vi "Washer Cluster Arrays ReadWrite.vi"(0 "Array Label":string(combo)="Aisle1", 1 "Write?":bool, 5 "configuration file path":path=path "C:/data/Washer Backup.ini", 7 "Program Execution":T1={"Test Fixture Hardware"={"Power "={"Yokogawa"={"WT210"={"Sample Rate (1: 0.25s)"=1, "A Range (12: 20A)"=11, "V Range (6: 600V)"=4, "Power VISA Yokogawa WT210"=""}, "WT500"={"Power VISA Yokogawa WT500"="", "V Range (8: 1000V)"=6, "I Range (7: 40A)"=7, "Update Rate (3: 500ms)"=2}}, "Aplus"={"Aplus IP Address"="192.168.1.101", "Remote Port"=502, "Instrument"="APLUS", "Instr Driver Revision"="1.03.0053"}, "Power Limits"={"Crest Factor"={"Upper Limit"=1.49, "Lower Limit"=1.34}, "Harmonic Content"={"Uthd"=2.0}, "Voltage"={"% Error"=2.0}, "Stability"={"<1 Watt "={"Wattage"=1.0, "Slope (mW/H)"=10.0}, ">1 Watt"={"1%Power/Hour"=1.0}}}, "Nominal Voltage"=120, "Time Limit (s)"=10800.0, "Power Variation Limit (%)"=50.0, "Power Supply"={"Chroma 61605"="CHROMA", "Use Chroma?"=FALSE}}, "Agilent 34972_1"="", "Hot Water Laurel"="", "Cold Water Laurel"="", "LV Program"=enum."DOE Stand", "MW100"="MW100", "Agilent 34972_2"="34972A_2", "Agilent 34972_3"="34972A_3", "IND560Scale"="MW100", "Avery Weigth Tronix Scale"={"IP Address"="", "Remote Port"=0}}, "GEA2"={"Address"=35, "Source"=228, "Viper/Hawk"=0}, "DOE Capacity Measurments"={"Weight 1"=35.0, "Model Number 1"="", "Temp 1"=0.0, "Serial Number 1"="", "Lab Number 1"="", "Lab Number 2"="", "Serial Number 2"="", "Temp 2"=0.0, "Model Number 2"="", "Weight 2"=0.0, "Lab Number 3"="", "Serial Number 3"="", "Temp 3"=0.0, "Model Number 3"="", "Weight 3"=0.0, "Lab Number 4"="", "Serial Number 4"="", "Temp 4"=0.0, "Model Number 4"="", "Weight 4"=0.0, "Capacity Measurment Output String"=[]}, "Appliance Details"={"Engineer:"="", "Model Number:"="", "Serial Number:"="", "Comments:"="", "Station ID:"="", "Technician:"="", "TR Number:"="", "Lab ID:"="", "Voltage:"="", "Water Pressure (PSI):"="", "FileVersionInfo"={"FileVersion"="", "ProductName"="", "InternalName"="", "CompanyName"="", "LegalCopyright"="", "FileDescription"=""}, "Test Date"="", "Computer Name"="", "IP Address"="", "Test Name"="", "Ambient RH:"="", "Supply Voltage"="", "Frequency:"="", "Build:"="", "Dishwasher Info"={"Open Cup Weight (gm):"=0.0, "Auto Cup Weight (gm):"=0.0, "Detergent:"="", "Inlet Temperature (F):"="", "Cycle Mode:"="", "Unit Control:"="", "Manufacturer:"=""}, "Washer Info"={"Hot Water Temperature (Fahrenheit)"="", "Cold Water Temperature (Fahrenheit)"="", "Capacity (cu.ft)"=0.0, "Initial Cloth Weight:"=0.0, "Cloth Lot:"=0, "Model Family"="", "Program Name"="", "Cycle Selection"="", "Wash Temperature"="", "Rinse Temperature"="", "Load Size"=""}, "File Name Output Array"=[], "Calibration Output Array"=[], "Filename"="", "Data File Paths"={"Data File Path"=path "", "Debug File Path"=path "", "Bus Log Path"=path ""}, "Test Type:"="", "Load Run #"=0}} {"GEA2"."Address" format="%x"; "GEA2"."Source" format="%x"; "GEA2"."Viper/Hawk" items=["Viper", "Hawk"]; "Test Fixture Hardware"."Power"."Yokogawa"."WT500"."Update Rate (3: 500ms)" items=["-", "100ms", "200ms", "500ms", "1s", "2s", "5s"]; "Test Fixture Hardware"."Power"."Yokogawa"."WT500"."I Range (7: 40A)" items=["AUTO", "500 mA", "1 A", "2 A", "5 A", "10 A", "20 A", "40 A", "S-AUTO", "50 mV", "100 mV", "200 mV", "500 mV", "1 V", "2 V", "5 V", "10 V", "250 mA", "500 mA", "1 A", "2.5 A", "5 A", "10 A", "20 A", "25 mV", "50 mV", "100 mV", "250 mV", "500 mV", "1 V", "2.5 V", "5 V"]; "Test Fixture Hardware"."Power"."Yokogawa"."WT500"."V Range (8: 1000V)" items=["AUTO", "15", "30", "60", "100", "150", "300", "600", "1000", "7.5", "15", "30", "50", "75", "150", "300", "500"]; "Test Fixture Hardware"."Power"."Yokogawa"."WT210"."V Range (6: 600V)" items=["Auto", "15V", "30V", "60V", "150V", "300V", "600V"]; "Test Fixture Hardware"."Power"."Yokogawa"."WT210"."A Range (12: 20A)" items=["Auto", "5mA", "10mA", "20mA", "50mA", "100mA", "200mA", "0.5A", "1A", "2A", "5A", "10A", "20A", "50mV", "100mV", "200mV", "2.5V", "5V", "10V"]; "Test Fixture Hardware"."Power"."Yokogawa"."WT210"."Sample Rate (1: 0.25s)" items=["0.1s", "0.25s", "0.5s", "1s", "2s", "5s"]}, 11 "error in (no error)":errorcluster) -> (4 "Output Cluster":T1={"Test Fixture Hardware"={"Power "={"Yokogawa"={"WT210"={"Sample Rate (1: 0.25s)"=1, "A Range (12: 20A)"=11, "V Range (6: 600V)"=4, "Power VISA Yokogawa WT210"=""}, "WT500"={"Power VISA Yokogawa WT500"="", "V Range (8: 1000V)"=6, "I Range (7: 40A)"=7, "Update Rate (3: 500ms)"=2}}, "Aplus"={"Aplus IP Address"="192.168.1.101", "Remote Port"=502, "Instrument"="APLUS", "Instr Driver Revision"="1.03.0053"}, "Power Limits"={"Crest Factor"={"Upper Limit"=1.49, "Lower Limit"=1.34}, "Harmonic Content"={"Uthd"=2.0}, "Voltage"={"% Error"=2.0}, "Stability"={"<1 Watt "={"Wattage"=1.0, "Slope (mW/H)"=10.0}, ">1 Watt"={"1%Power/Hour"=1.0}}}, "Nominal Voltage"=120, "Time Limit (s)"=10800.0, "Power Variation Limit (%)"=50.0, "Power Supply"={"Chroma 61605"="CHROMA", "Use Chroma?"=FALSE}}, "Agilent 34972_1"="", "Hot Water Laurel"="", "Cold Water Laurel"="", "LV Program"=enum."DOE Stand", "MW100"="MW100", "Agilent 34972_2"="34972A_2", "Agilent 34972_3"="34972A_3", "IND560Scale"="MW100", "Avery Weigth Tronix Scale"={"IP Address"="", "Remote Port"=0}}, "GEA2"={"Address"=35, "Source"=228, "Viper/Hawk"=0}, "DOE Capacity Measurments"={"Weight 1"=35.0, "Model Number 1"="", "Temp 1"=0.0, "Serial Number 1"="", "Lab Number 1"="", "Lab Number 2"="", "Serial Number 2"="", "Temp 2"=0.0, "Model Number 2"="", "Weight 2"=0.0, "Lab Number 3"="", "Serial Number 3"="", "Temp 3"=0.0, "Model Number 3"="", "Weight 3"=0.0, "Lab Number 4"="", "Serial Number 4"="", "Temp 4"=0.0, "Model Number 4"="", "Weight 4"=0.0, "Capacity Measurment Output String"=[]}, "Appliance Details"={"Engineer:"="", "Model Number:"="", "Serial Number:"="", "Comments:"="", "Station ID:"="", "Technician:"="", "TR Number:"="", "Lab ID:"="", "Voltage:"="", "Water Pressure (PSI):"="", "FileVersionInfo"={"FileVersion"="", "ProductName"="", "InternalName"="", "CompanyName"="", "LegalCopyright"="", "FileDescription"=""}, "Test Date"="", "Computer Name"="", "IP Address"="", "Test Name"="", "Ambient RH:"="", "Supply Voltage"="", "Frequency:"="", "Build:"="", "Dishwasher Info"={"Open Cup Weight (gm):"=0.0, "Auto Cup Weight (gm):"=0.0, "Detergent:"="", "Inlet Temperature (F):"="", "Cycle Mode:"="", "Unit Control:"="", "Manufacturer:"=""}, "Washer Info"={"Hot Water Temperature (Fahrenheit)"="", "Cold Water Temperature (Fahrenheit)"="", "Capacity (cu.ft)"=0.0, "Initial Cloth Weight:"=0.0, "Cloth Lot:"=0, "Model Family"="", "Program Name"="", "Cycle Selection"="", "Wash Temperature"="", "Rinse Temperature"="", "Load Size"=""}, "File Name Output Array"=[], "Calibration Output Array"=[], "Filename"="", "Data File Paths"={"Data File Path"=path "", "Debug File Path"=path "", "Bus Log Path"=path ""}, "Test Type:"="", "Load Run #"=0}} {"GEA2"."Address" format="%x"; "GEA2"."Source" format="%x"; "GEA2"."Viper/Hawk" items=["Viper", "Hawk"]; "Test Fixture Hardware"."Power"."Yokogawa"."WT500"."Update Rate (3: 500ms)" items=["-", "100ms", "200ms", "500ms", "1s", "2s", "5s"]; "Test Fixture Hardware"."Power"."Yokogawa"."WT500"."I Range (7: 40A)" items=["AUTO", "500 mA", "1 A", "2 A", "5 A", "10 A", "20 A", "40 A", "S-AUTO", "50 mV", "100 mV", "200 mV", "500 mV", "1 V", "2 V", "5 V", "10 V", "250 mA", "500 mA", "1 A", "2.5 A", "5 A", "10 A", "20 A", "25 mV", "50 mV", "100 mV", "250 mV", "500 mV", "1 V", "2.5 V", "5 V"]; "Test Fixture Hardware"."Power"."Yokogawa"."WT500"."V Range (8: 1000V)" items=["AUTO", "15", "30", "60", "100", "150", "300", "600", "1000", "7.5", "15", "30", "50", "75", "150", "300", "500"]; "Test Fixture Hardware"."Power"."Yokogawa"."WT210"."V Range (6: 600V)" items=["Auto", "15V", "30V", "60V", "150V", "300V", "600V"]; "Test Fixture Hardware"."Power"."Yokogawa"."WT210"."A Range (12: 20A)" items=["Auto", "5mA", "10mA", "20mA", "50mA", "100mA", "200mA", "0.5A", "1A", "2A", "5A", "10A", "20A", "50mV", "100mV", "200mV", "2.5V", "5V", "10V"]; "Test Fixture Hardware"."Power"."Yokogawa"."WT210"."Sample Rate (1: 0.25s)" items=["0.1s", "0.25s", "0.5s", "1s", "2s", "5s"]}, 6 "Local Control?":bool, 15 "error out":errorcluster)   [LabVIEW 2014]
uses:
  Type Definitions/DOE Main Control.ctl
  Type Definitions/DOE Test Fixture Hardware.ctl
  Utility/Type Definitions/UTILITY Power Inputs Control.ctl
  Utility/Save File/File Setup (Public)/Type Definition/Save File DOE LabView Program.ctl
  Drivers/Avery Weight Tronix/Type Definitions/Avery Weight Tronix IP Address.ctl
  GEA2.ctl
  Type Definitions/DOE Capacity Measurments.ctl
  Utility/Save File/File Setup (Public)/Type Definition/Save File DISH Dishwasher Details.ctl
  <vilib>/Platform/fileVersionInfo.llb/FileVersionInformation.ctl
  Utility/Save File/File Setup (Public)/Type Definition/Save File DOE Data Save Filepaths.ctl
  <vilib>/Utility/config.llb/Write Key (Double).vi
  <vilib>/Utility/config.llb/Write Key (String).vi
  <vilib>/Utility/config.llb/Write Key (Path).vi
  <vilib>/Utility/config.llb/Write Key (I32).vi
  <vilib>/Utility/config.llb/Write Key (U32).vi
  <vilib>/Utility/config.llb/Write Key (Boolean).vi
  <vilib>/Utility/config.llb/Read Key (Double).vi
  <vilib>/Utility/config.llb/Read Key (String).vi
  <vilib>/Utility/config.llb/Read Key (Path).vi
  <vilib>/Utility/config.llb/Read Key (I32).vi
  <vilib>/Utility/config.llb/Read Key (U32).vi
  <vilib>/Utility/config.llb/Read Key (Boolean).vi
  <vilib>/Utility/config.llb/NI_LVConfig.lvlib
  <vilib>/Utility/VariantDataType/VariantType.lvlib
  Utility/Save File/File Setup.lvlib
panel:
  in  "Local Execution":T1={"Test Fixture Hardware"={"Power "={"Yokogawa"={"WT210"={"Sample Rate (1: 0.25s)"=1, "A Range (12: 20A)"=11, "V Range (6: 600V)"=4, "Power VISA Yokogawa WT210"=""}, "WT500"={"Power VISA Yokogawa WT500"="", "V Range (8: 1000V)"=6, "I Range (7: 40A)"=7, "Update Rate (3: 500ms)"=2}}, "Aplus"={"Aplus IP Address"="192.168.1.101", "Remote Port"=502, "Instrument"="APLUS", "Instr Driver Revision"="1.03.0053"}, "Power Limits"={"Crest Factor"={"Upper Limit"=1.49, "Lower Limit"=1.34}, "Harmonic Content"={"Uthd"=2.0}, "Voltage"={"% Error"=2.0}, "Stability"={"<1 Watt "={"Wattage"=1.0, "Slope (mW/H)"=10.0}, ">1 Watt"={"1%Power/Hour"=1.0}}}, "Nominal Voltage"=120, "Time Limit (s)"=10800.0, "Power Variation Limit (%)"=50.0, "Power Supply"={"Chroma 61605"="CHROMA", "Use Chroma?"=FALSE}}, "Agilent 34972_1"="", "Hot Water Laurel"="", "Cold Water Laurel"="", "LV Program"=enum."DOE Stand", "MW100"="MW100", "Agilent 34972_2"="34972A_2", "Agilent 34972_3"="34972A_3", "IND560Scale"="MW100", "Avery Weigth Tronix Scale"={"IP Address"="", "Remote Port"=0}}, "GEA2"={"Address"=35, "Source"=228, "Viper/Hawk"=0}, "DOE Capacity Measurments"={"Weight 1"=35.0, "Model Number 1"="", "Temp 1"=0.0, "Serial Number 1"="", "Lab Number 1"="", "Lab Number 2"="", "Serial Number 2"="", "Temp 2"=0.0, "Model Number 2"="", "Weight 2"=0.0, "Lab Number 3"="", "Serial Number 3"="", "Temp 3"=0.0, "Model Number 3"="", "Weight 3"=0.0, "Lab Number 4"="", "Serial Number 4"="", "Temp 4"=0.0, "Model Number 4"="", "Weight 4"=0.0, "Capacity Measurment Output String"=[]}, "Appliance Details"={"Engineer:"="", "Model Number:"="", "Serial Number:"="", "Comments:"="", "Station ID:"="", "Technician:"="", "TR Number:"="", "Lab ID:"="", "Voltage:"="", "Water Pressure (PSI):"="", "FileVersionInfo"={"FileVersion"="", "ProductName"="", "InternalName"="", "CompanyName"="", "LegalCopyright"="", "FileDescription"=""}, "Test Date"="", "Computer Name"="", "IP Address"="", "Test Name"="", "Ambient RH:"="", "Supply Voltage"="", "Frequency:"="", "Build:"="", "Dishwasher Info"={"Open Cup Weight (gm):"=0.0, "Auto Cup Weight (gm):"=0.0, "Detergent:"="", "Inlet Temperature (F):"="", "Cycle Mode:"="", "Unit Control:"="", "Manufacturer:"=""}, "Washer Info"={"Hot Water Temperature (Fahrenheit)"="", "Cold Water Temperature (Fahrenheit)"="", "Capacity (cu.ft)"=0.0, "Initial Cloth Weight:"=0.0, "Cloth Lot:"=0, "Model Family"="", "Program Name"="", "Cycle Selection"="", "Wash Temperature"="", "Rinse Temperature"="", "Load Size"=""}, "File Name Output Array"=[], "Calibration Output Array"=[], "Filename"="", "Data File Paths"={"Data File Path"=path "", "Debug File Path"=path "", "Bus Log Path"=path ""}, "Test Type:"="", "Load Run #"=0}} {"GEA2"."Address" format="%x"; "GEA2"."Source" format="%x"; "GEA2"."Viper/Hawk" items=["Viper", "Hawk"]; "Test Fixture Hardware"."Power"."Yokogawa"."WT500"."Update Rate (3: 500ms)" items=["-", "100ms", "200ms", "500ms", "1s", "2s", "5s"]; "Test Fixture Hardware"."Power"."Yokogawa"."WT500"."I Range (7: 40A)" items=["AUTO", "500 mA", "1 A", "2 A", "5 A", "10 A", "20 A", "40 A", "S-AUTO", "50 mV", "100 mV", "200 mV", "500 mV", "1 V", "2 V", "5 V", "10 V", "250 mA", "500 mA", "1 A", "2.5 A", "5 A", "10 A", "20 A", "25 mV", "50 mV", "100 mV", "250 mV", "500 mV", "1 V", "2.5 V", "5 V"]; "Test Fixture Hardware"."Power"."Yokogawa"."WT500"."V Range (8: 1000V)" items=["AUTO", "15", "30", "60", "100", "150", "300", "600", "1000", "7.5", "15", "30", "50", "75", "150", "300", "500"]; "Test Fixture Hardware"."Power"."Yokogawa"."WT210"."V Range (6: 600V)" items=["Auto", "15V", "30V", "60V", "150V", "300V", "600V"]; "Test Fixture Hardware"."Power"."Yokogawa"."WT210"."A Range (12: 20A)" items=["Auto", "5mA", "10mA", "20mA", "50mA", "100mA", "200mA", "0.5A", "1A", "2A", "5A", "10A", "20A", "50mV", "100mV", "200mV", "2.5V", "5V", "10V"]; "Test Fixture Hardware"."Power"."Yokogawa"."WT210"."Sample Rate (1: 0.25s)" items=["0.1s", "0.25s", "0.5s", "1s", "2s", "5s"]}
  in  "Washer Variable":T1={"Test Fixture Hardware"={"Power "={"Yokogawa"={"WT210"={"Sample Rate (1: 0.25s)"=1, "A Range (12: 20A)"=11, "V Range (6: 600V)"=4, "Power VISA Yokogawa WT210"=""}, "WT500"={"Power VISA Yokogawa WT500"="", "V Range (8: 1000V)"=6, "I Range (7: 40A)"=7, "Update Rate (3: 500ms)"=2}}, "Aplus"={"Aplus IP Address"="192.168.1.101", "Remote Port"=502, "Instrument"="APLUS", "Instr Driver Revision"="1.03.0053"}, "Power Limits"={"Crest Factor"={"Upper Limit"=1.49, "Lower Limit"=1.34}, "Harmonic Content"={"Uthd"=2.0}, "Voltage"={"% Error"=2.0}, "Stability"={"<1 Watt "={"Wattage"=1.0, "Slope (mW/H)"=10.0}, ">1 Watt"={"1%Power/Hour"=1.0}}}, "Nominal Voltage"=120, "Time Limit (s)"=10800.0, "Power Variation Limit (%)"=50.0, "Power Supply"={"Chroma 61605"="CHROMA", "Use Chroma?"=FALSE}}, "Agilent 34972_1"="", "Hot Water Laurel"="", "Cold Water Laurel"="", "LV Program"=enum."DOE Stand", "MW100"="MW100", "Agilent 34972_2"="34972A_2", "Agilent 34972_3"="34972A_3", "IND560Scale"="MW100", "Avery Weigth Tronix Scale"={"IP Address"="", "Remote Port"=0}}, "GEA2"={"Address"=35, "Source"=228, "Viper/Hawk"=0}, "DOE Capacity Measurments"={"Weight 1"=35.0, "Model Number 1"="", "Temp 1"=0.0, "Serial Number 1"="", "Lab Number 1"="", "Lab Number 2"="", "Serial Number 2"="", "Temp 2"=0.0, "Model Number 2"="", "Weight 2"=0.0, "Lab Number 3"="", "Serial Number 3"="", "Temp 3"=0.0, "Model Number 3"="", "Weight 3"=0.0, "Lab Number 4"="", "Serial Number 4"="", "Temp 4"=0.0, "Model Number 4"="", "Weight 4"=0.0, "Capacity Measurment Output String"=[]}, "Appliance Details"={"Engineer:"="", "Model Number:"="", "Serial Number:"="", "Comments:"="", "Station ID:"="", "Technician:"="", "TR Number:"="", "Lab ID:"="", "Voltage:"="", "Water Pressure (PSI):"="", "FileVersionInfo"={"FileVersion"="", "ProductName"="", "InternalName"="", "CompanyName"="", "LegalCopyright"="", "FileDescription"=""}, "Test Date"="", "Computer Name"="", "IP Address"="", "Test Name"="", "Ambient RH:"="", "Supply Voltage"="", "Frequency:"="", "Build:"="", "Dishwasher Info"={"Open Cup Weight (gm):"=0.0, "Auto Cup Weight (gm):"=0.0, "Detergent:"="", "Inlet Temperature (F):"="", "Cycle Mode:"="", "Unit Control:"="", "Manufacturer:"=""}, "Washer Info"={"Hot Water Temperature (Fahrenheit)"="", "Cold Water Temperature (Fahrenheit)"="", "Capacity (cu.ft)"=0.0, "Initial Cloth Weight:"=0.0, "Cloth Lot:"=0, "Model Family"="", "Program Name"="", "Cycle Selection"="", "Wash Temperature"="", "Rinse Temperature"="", "Load Size"=""}, "File Name Output Array"=[], "Calibration Output Array"=[], "Filename"="", "Data File Paths"={"Data File Path"=path "", "Debug File Path"=path "", "Bus Log Path"=path ""}, "Test Type:"="", "Load Run #"=0}} {"GEA2"."Address" format="%x"; "GEA2"."Source" format="%x"; "GEA2"."Viper/Hawk" items=["Viper", "Hawk"]; "Test Fixture Hardware"."Power"."Yokogawa"."WT500"."Update Rate (3: 500ms)" items=["-", "100ms", "200ms", "500ms", "1s", "2s", "5s"]; "Test Fixture Hardware"."Power"."Yokogawa"."WT500"."I Range (7: 40A)" items=["AUTO", "500 mA", "1 A", "2 A", "5 A", "10 A", "20 A", "40 A", "S-AUTO", "50 mV", "100 mV", "200 mV", "500 mV", "1 V", "2 V", "5 V", "10 V", "250 mA", "500 mA", "1 A", "2.5 A", "5 A", "10 A", "20 A", "25 mV", "50 mV", "100 mV", "250 mV", "500 mV", "1 V", "2.5 V", "5 V"]; "Test Fixture Hardware"."Power"."Yokogawa"."WT500"."V Range (8: 1000V)" items=["AUTO", "15", "30", "60", "100", "150", "300", "600", "1000", "7.5", "15", "30", "50", "75", "150", "300", "500"]; "Test Fixture Hardware"."Power"."Yokogawa"."WT210"."V Range (6: 600V)" items=["Auto", "15V", "30V", "60V", "150V", "300V", "600V"]; "Test Fixture Hardware"."Power"."Yokogawa"."WT210"."A Range (12: 20A)" items=["Auto", "5mA", "10mA", "20mA", "50mA", "100mA", "200mA", "0.5A", "1A", "2A", "5A", "10A", "20A", "50mV", "100mV", "200mV", "2.5V", "5V", "10V"]; "Test Fixture Hardware"."Power"."Yokogawa"."WT210"."Sample Rate (1: 0.25s)" items=["0.1s", "0.25s", "0.5s", "1s", "2s", "5s"]}
  out "String array out":string="[1,23-2-3]\n[4-3,22-2]\n[3-4,01-8]\n[0-7-6,66]"
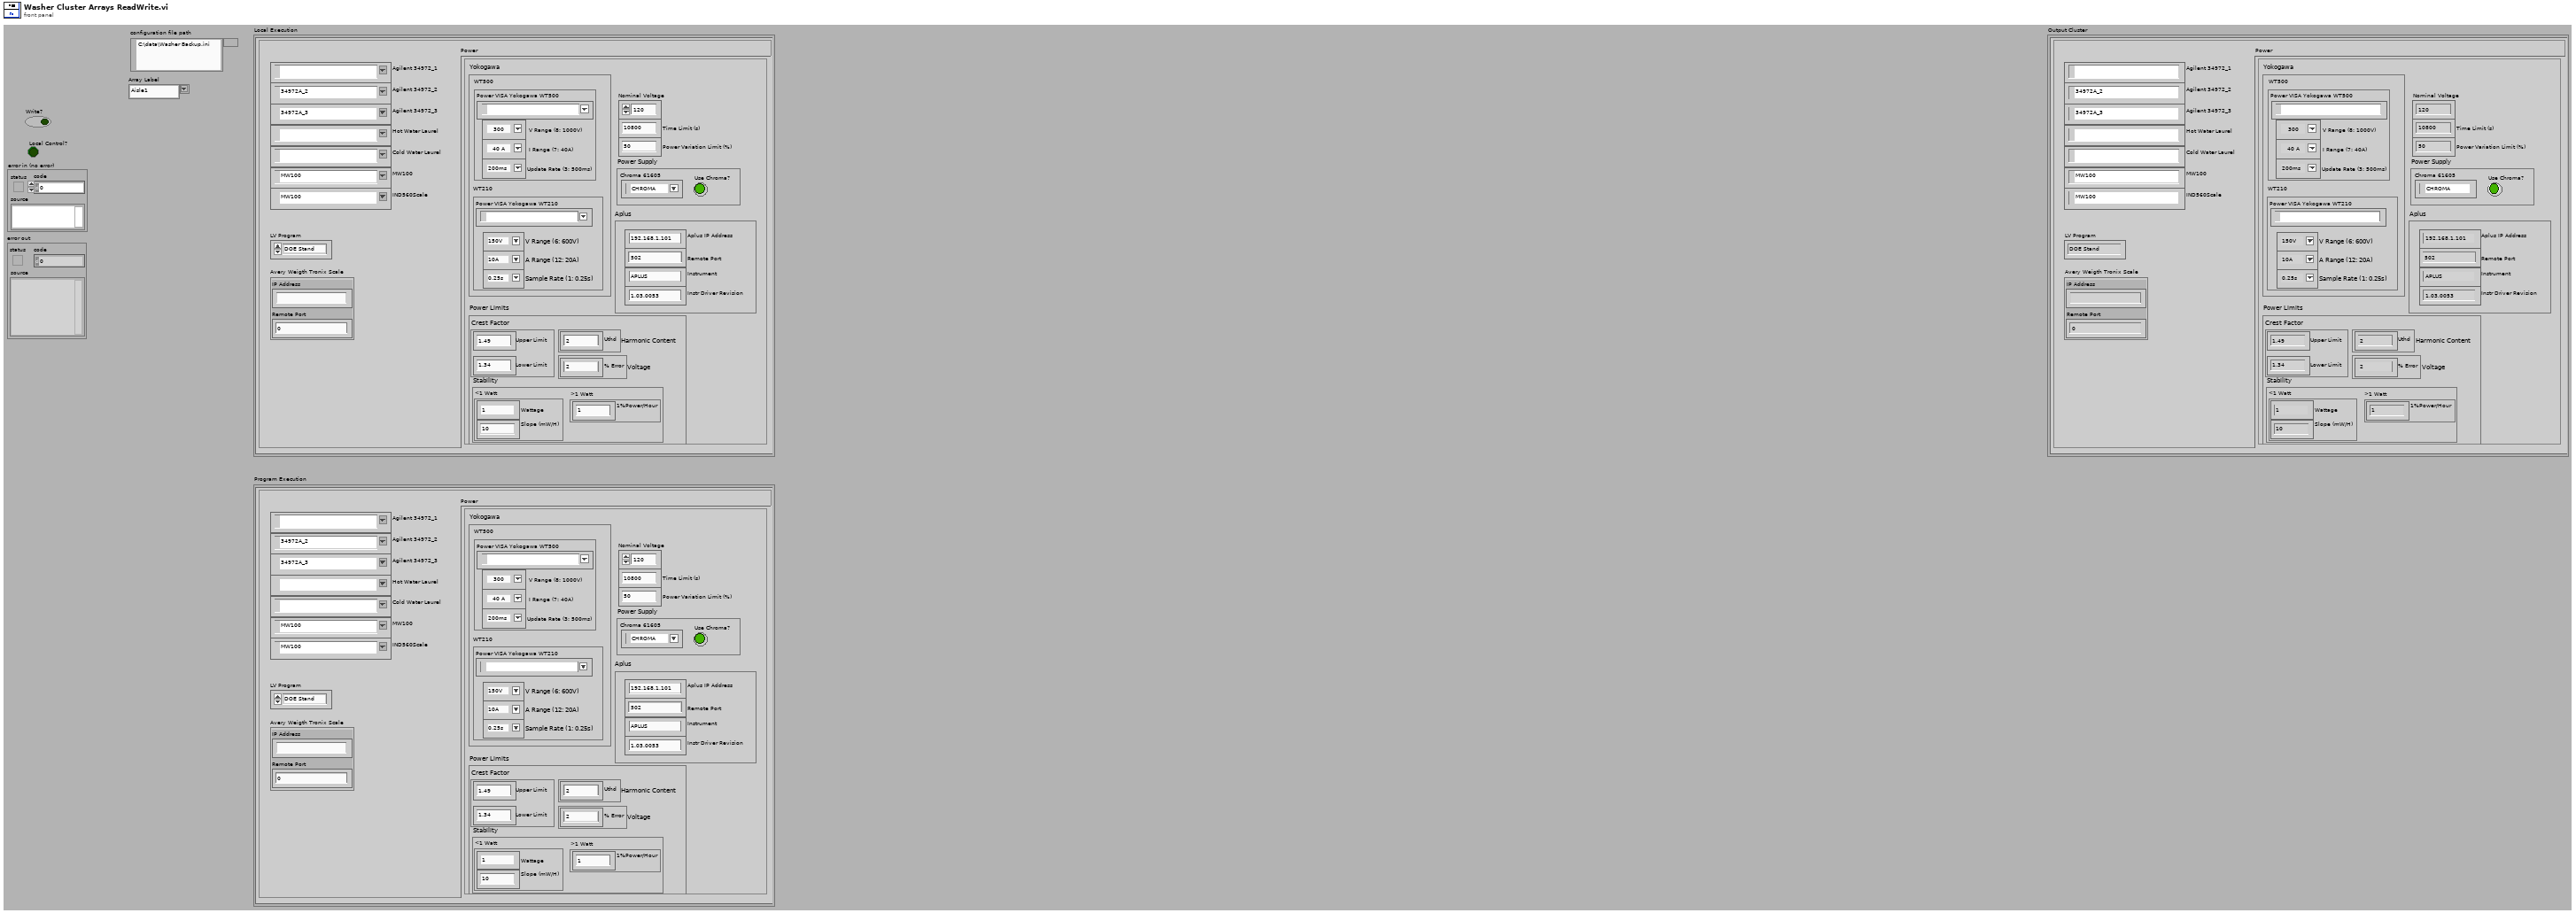
[diagram p1: front panel]
types:
  T1 = typedef "DOE Main Control.ctl" = cluster{"Test Fixture Hardware":T2, "GEA2":T6, "DOE Capacity Measurments":T7, "Appliance Details":T8}
  T2 = typedef "DOE Test Fixture Hardware.ctl" = cluster{"Power ":T3, "Agilent 34972_1":refnum<visa-resource-name>, "Hot Water Laurel":refnum<visa-resource-name>, "Cold Water Laurel":refnum<visa-resource-name>, "LV Program":T4, "MW100":refnum<visa-resource-name>, "Agilent 34972_2":refnum<visa-resource-name>, "Agilent 34972_3":refnum<visa-resource-name>, "IND560Scale":refnum<visa-resource-name>, "Avery Weigth Tronix Scale":T5}
  T3 = typedef "UTILITY Power Inputs Control.ctl" = cluster{"Yokogawa":cluster{"WT210":cluster{"Sample Rate (1: 0.25s)":i32, "A Range (12: 20A)":i32, "V Range (6: 600V)":i32, "Power VISA Yokogawa WT210":refnum<visa-resource-name>}, "WT500":cluster{"Power VISA Yokogawa WT500":refnum<visa-resource-name>, "V Range (8: 1000V)":i32, "I Range (7: 40A)":i32, "Update Rate (3: 500ms)":i32}}, "Aplus":cluster{"Aplus IP Address":string, "Remote Port":i32, "Instrument":string, "Instr Driver Revision":string}, "Power Limits":cluster{"Crest Factor":cluster{"Upper Limit":dbl, "Lower Limit":dbl}, "Harmonic Content":cluster{"Uthd":dbl}, "Voltage":cluster{"% Error":dbl}, "Stability":cluster{"<1 Watt ":cluster{"Wattage":dbl, "Slope (mW/H)":dbl}, ">1 Watt":cluster{"1%Power/Hour":dbl}}}, "Nominal Voltage":i32, "Time Limit (s)":dbl, "Power Variation Limit (%)":dbl, "Power Supply":cluster{"Chroma 61605":refnum<visa-resource-name>, "Use Chroma?":bool}}
  T4 = typedef "File Setup.lvlib/Save File DOE LabView Program.ctl" = enum16{"DOE Stand", "Dishwasher Kitchen", "Portable Stand", "UL Left", "UL Right"}
  T5 = typedef "Avery Weight Tronix IP Address.ctl" = cluster{"IP Address":string, "Remote Port":u16}
  T6 = typedef "GEA2.ctl" = cluster{"Address":u8, "Source":u8, "Viper/Hawk":u8}
  T7 = typedef "DOE Capacity Measurments.ctl" = cluster{"Weight 1":dbl, "Model Number 1":string, "Temp 1":dbl, "Serial Number 1":string, "Lab Number 1":string, "Lab Number 2":string, "Serial Number 2":string, "Temp 2":dbl, "Model Number 2":string, "Weight 2":dbl, "Lab Number 3":string, "Serial Number 3":string, "Temp 3":dbl, "Model Number 3":string, "Weight 3":dbl, "Lab Number 4":string, "Serial Number 4":string, "Temp 4":dbl, "Model Number 4":string, "Weight 4":dbl, "Capacity Measurment Output String":string[][]}
  T8 = typedef "File Setup.lvlib/Save File DISH Dishwasher Details.ctl" = cluster{"Engineer:":string, "Model Number:":string, "Serial Number:":string, "Comments:":string, "Station ID:":string, "Technician:":string, "TR Number:":string, "Lab ID:":string, "Voltage:":string, "Water Pressure (PSI):":string, "FileVersionInfo":T9, "Test Date":string, "Computer Name":string, "IP Address":string, "Test Name":string, "Ambient RH:":string, "Supply Voltage":string, "Frequency:":string, "Build:":string, "Dishwasher Info":cluster{"Open Cup Weight (gm):":dbl, "Auto Cup Weight (gm):":dbl, "Detergent:":string, "Inlet Temperature (F):":string, "Cycle Mode:":string, "Unit Control:":string, "Manufacturer:":string}, "Washer Info":cluster{"Hot Water Temperature (Fahrenheit)":string, "Cold Water Temperature (Fahrenheit)":string, "Capacity (cu.ft)":dbl, "Initial Cloth Weight:":dbl, "Cloth Lot:":i32, "Model Family":string, "Program Name":string, "Cycle Selection":string, "Wash Temperature":string, "Rinse Temperature":string, "Load Size":string}, "File Name Output Array":string[][], "Calibration Output Array":string[][], "Filename":string, "Data File Paths":T10, "Test Type:":string, "Load Run #":i32}
  T9 = typedef "FileVersionInformation.ctl" = cluster{"FileVersion":string, "ProductName":string, "InternalName":string, "CompanyName":string, "LegalCopyright":string, "FileDescription":string}
  T10 = typedef "File Setup.lvlib/Save File DOE Data Save Filepaths.ctl" = cluster{"Data File Path":path, "Debug File Path":path, "Bus Log Path":path}
  T11 = typedef "NI_LVConfig.lvlib/Config Data RefNum.ctl" = refnum<k1>
  T12 = typedef "VariantType.lvlib/Type.ctl" = enum8{"Invalid Type", "Void", "I8", "I16", "I32", "I64", "U8", "U16", "U32", "U64", "Single Float", "Double Float", "Extended Float", "Single Complex", "Double Complex", "Extended Complex", "Enum U8", "Enum U16", "Enum U32", "Enum U64", "Single Float With Unit", "Double Float With Unit", "Extended Float With Unit", "Single Complex with Unit", "Double Complex with Unit", "Extended Complex with Unit", "Boolean", "String", "Path", "Picture", "Tag", "Array", "Cluster", "Variant", "LV Variant", "Waveform", "Timestamp", "Digital Waveform", "Digital Data", "ExpressData", "Refnum", "External Data", "VI", "Poly VI", "LabVIEW Class Instance", "Fixed Point"}
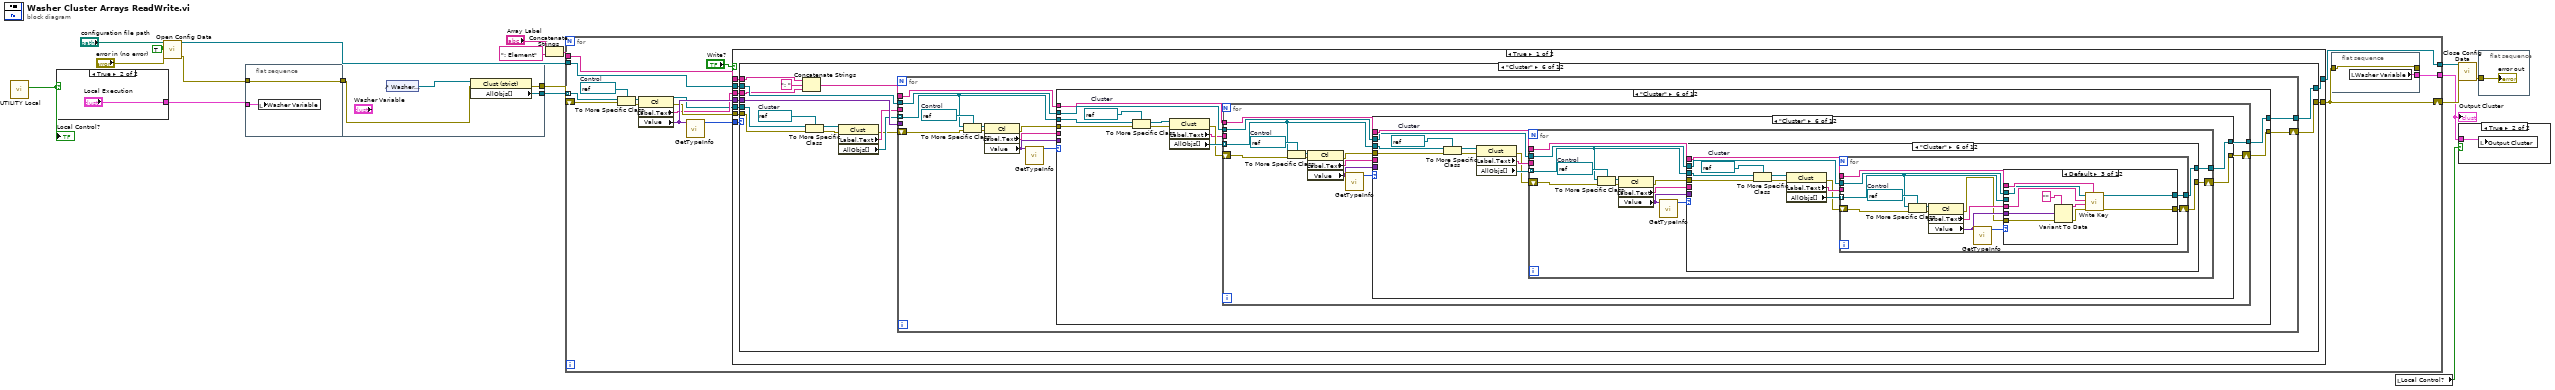
[diagram p0: block diagram]
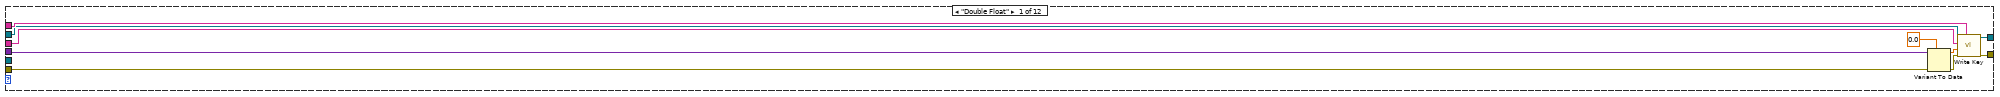
[diagram p2: hidden frame]
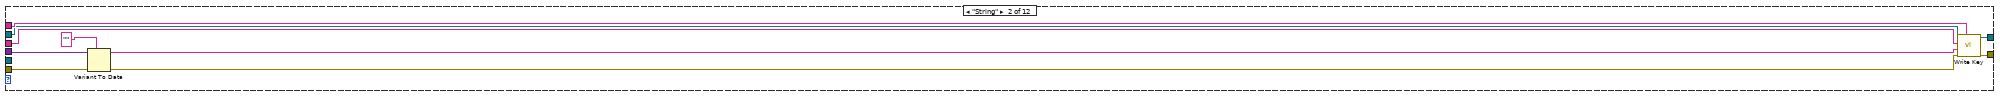
[diagram p3: hidden frame]
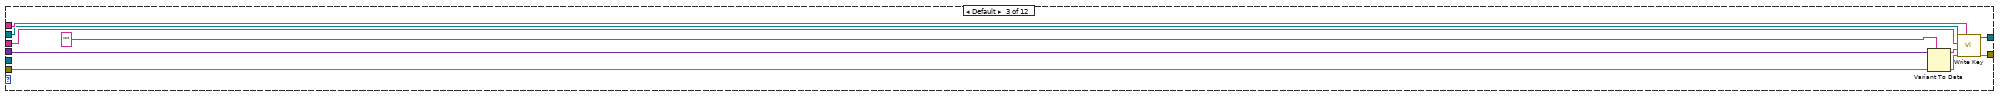
[diagram p4: hidden frame]
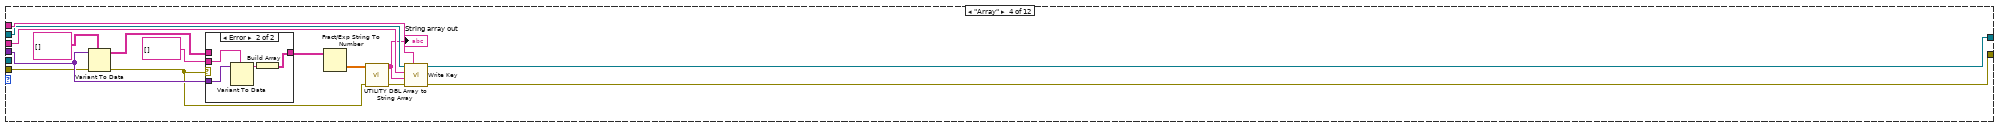
[diagram p5: hidden frame]
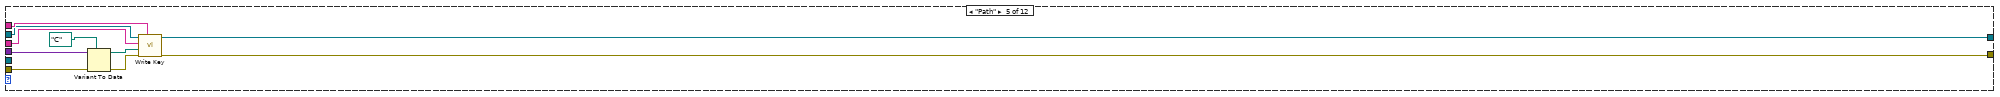
[diagram p7: hidden frame]
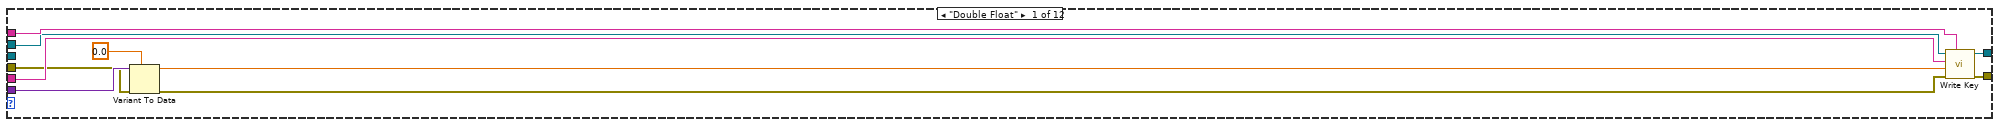
[diagram p8: hidden frame]
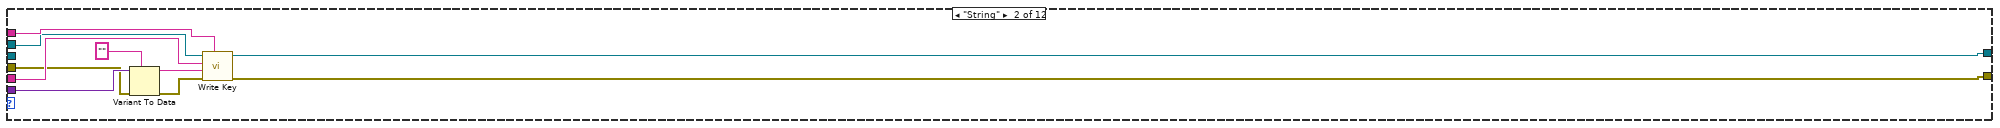
[diagram p9: hidden frame]
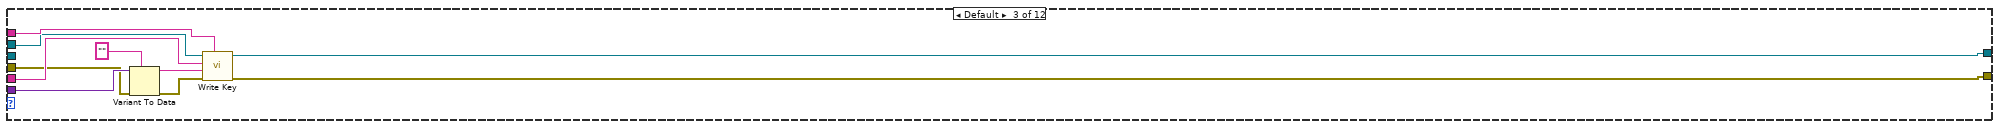
[diagram p10: hidden frame]
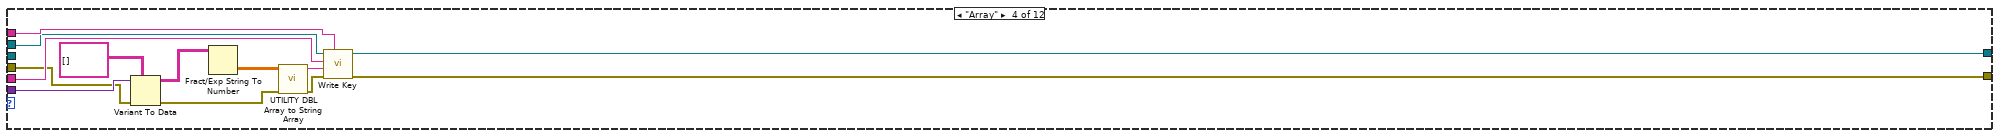
[diagram p11: hidden frame]
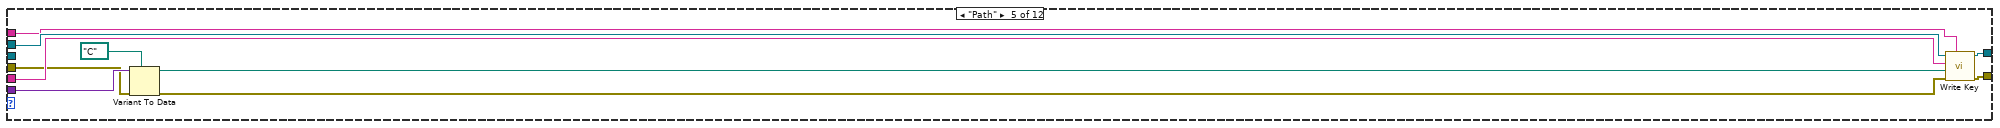
[diagram p12: hidden frame]
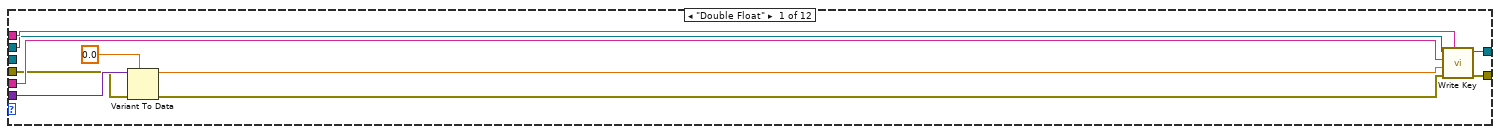
[diagram p13: hidden frame]
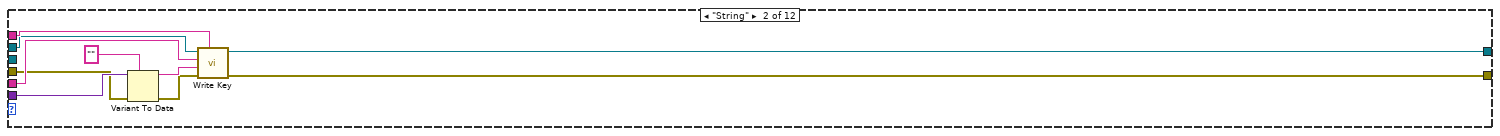
[diagram p14: hidden frame]
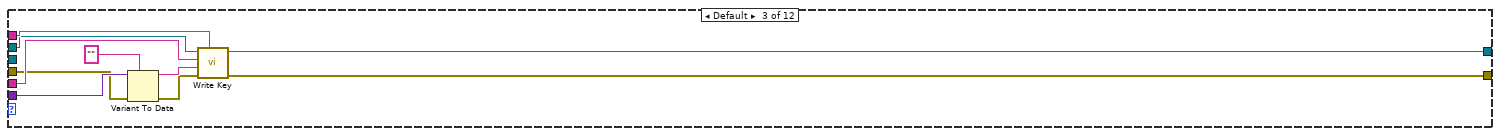
[diagram p15: hidden frame]
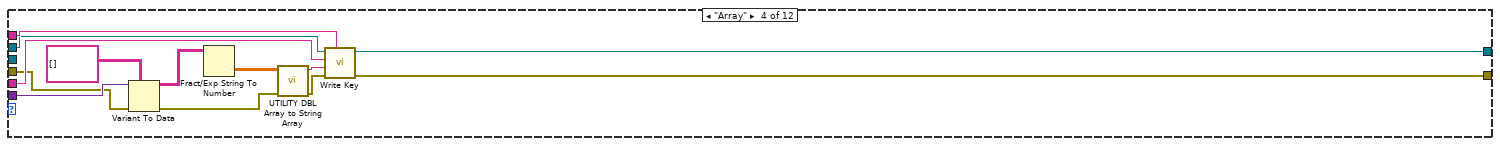
[diagram p16: hidden frame]
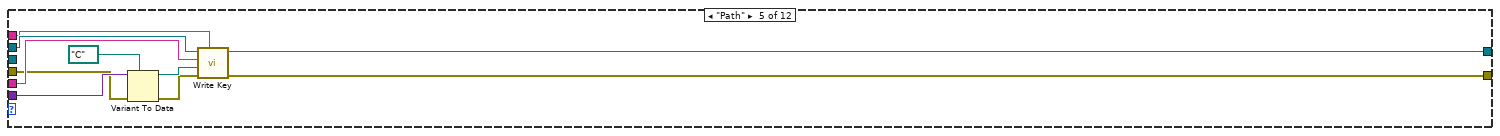
[diagram p17: hidden frame]
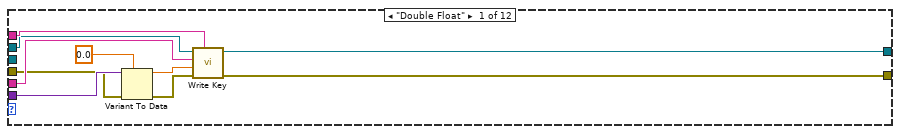
[diagram p18: hidden frame]
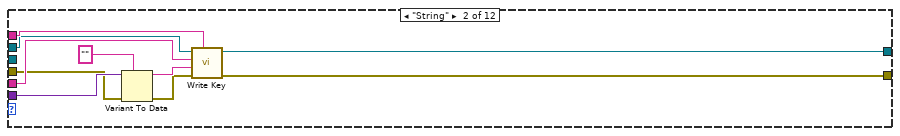
[diagram p19: hidden frame]
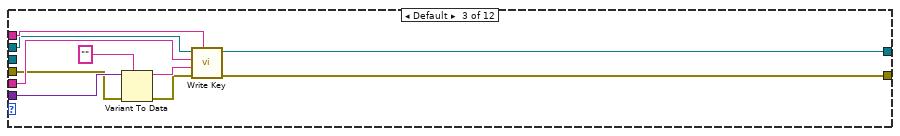
[diagram p20: hidden frame]
diagram:
  n1 = call "UTILITY Local.vi"() -> ("Local?"=w6:bool)  [unwired: 11 in]
  "Local Control?" <- w6
  n2 = case shown="True" w6 {
    tunnel: ["Program Execution" "Local Execution"] -> w8
    frame False {
    }
    frame True {
    }
  }
  n3 = call <vilib>:"Open Config Data.vi"("error in (no error)"="error in (no error)", "create file if necessary (T)"=TRUE, "configuration file path"="configuration file path") -> ("error out"=w14:errorcluster, "refnum"=w16:T11)  [unwired: 6 in, 1 out]
  n4 = flat-sequence {
    tunnel: w14 -> [w22]
    tunnel: [w22] -> w5
    tunnel: w8 -> [w21]
    tunnel: [w26] -> w4
    tunnel: [w24] -> w3
    tunnel: w5 -> [w25]
    frame #0 {
      n5 = local write "Washer Variable"(w21) -> ()
    }
    frame #1 {
      n6 = control-ref of="Washer Variable"() -> (w23:refnum<vi>)
      n7 = property class="Clust (strict)"(reference=w23, error in=w25) -> (error out=w24:errorcluster, "AllObjs[]"=w26:refnum<vi>[])  [unwired: 1 out]
    }
  }
  n8 = Concatenate Strings("Array Label", ": Element" ("string")) -> (w1:string)
  n9 = for {
    tunnel: w4 -> [w42] mode=indexing
    tunnel: w16 -> [w40]
    tunnel: [w39] -> w9
    shift-right: [w30] -> w10
    shift-left: w3 -> [w38]
    tunnel: w1 -> [w31]
    tunnel: [w29] -> w2
    w41 = refnum<vi> refnum  # Control
    n10 = To More Specific Class(target class=w41, reference=w42, error in=w38) -> (specific class reference=w27:refnum<vi>, error out=w33:errorcluster)
    n11 = property class="Ctl"(reference=w27, error in=w33) -> (reference out=w28:refnum<vi>, error out=w34:errorcluster, "Label.Text"=w32:string, "Value"=w35:variant)
    n12 = call <vilib>:"GetTypeInfo.vi"("Variant"=w35) -> ("Type Enum"=w36:T12)  [unwired: 6 in, 4 out]
    n13 = case shown="True" "Write?" {
      tunnel: w31 -> [w53 w755]
      tunnel: w32 -> [w52 w754]
      tunnel: w35 -> [w51 w752]
      tunnel: w40 -> [w50 w751]
      tunnel: [w49 w748] -> w30
      tunnel: [w48 w749] -> w39
      tunnel: w28 -> [w45 w750]
      tunnel: w36 -> [w47 w747]
      tunnel: w34 -> [w46 w753]
      frame True {
        n14 = case shown="\"Cluster\"" w47 {
          tunnel: w53 -> [w63 w73 w83 w98 w113 w117 w695 w705 w716 w726 w734 w744]
          tunnel: w52 -> [w62 w72 w82 w97 w112 w116 w694 w704 w715 w725 w731 w742]
          tunnel: w51 -> [w61 w71 w81 w90 w111 w125 w693 w703 w714 w724 w733 w741]
          tunnel: w50 -> [w60 w70 w80 w96 w110 w119 w692 w702 w713 w723 w732 w743]
          tunnel: [w59 w69 w79 w95 w109 w123 w691 w701 w712 w722 w729 w739] -> w49
          tunnel: [w58 w68 w78 w94 w108 w124 w690 w700 w711 w721 w730 w740] -> w48
          tunnel: w46 -> [w55 w64 w75 w86 w105 w126 w687 w697 w707 w718 w728 w738]
          tunnel: w45 -> [_ _ _ _ _ w121 _ _ _ _ _ _]
          frame "Double Float" {
            n15 = Variant To Data(error in=w55, type=0.0, Variant=w61) -> (data=w57:dbl, error out=w54:errorcluster)
            n16 = call-poly <vilib>:"Write Key.vi"("section"=w63, "error in (no error)"=w54, "value"=w57, "key"=w62, "refnum"=w60) -> ("error out"=w59:errorcluster, "refnum out"=w58:T11)  [unwired: 4 in, 1 out]
          }
          frame "String" {
            n17 = Variant To Data(error in=w64, type="" ("Label.Text"), Variant=w71) -> (data=w67:string, error out=w65:errorcluster)
            n18 = call-poly <vilib>:"Write Key.vi"("section"=w73, "error in (no error)"=w65, "value"=w67, "key"=w72, "refnum"=w70) -> ("error out"=w69:errorcluster, "refnum out"=w68:T11)  [unwired: 4 in, 1 out]
          }
          frame Default {
            n19 = Variant To Data(error in=w75, type="" ("Label.Text"), Variant=w81) -> (data=w77:string, error out=w74:errorcluster)
            n20 = call-poly <vilib>:"Write Key.vi"("section"=w83, "error in (no error)"=w74, "value"=w77, "key"=w82, "refnum"=w80) -> ("error out"=w79:errorcluster, "refnum out"=w78:T11)  [unwired: 4 in, 1 out]
          }
          frame "Array" {
            n21 = Variant To Data(error in=w86, type=string[][] [], Variant=w90) -> (data=w92:string[][], error out=w85:errorcluster)
            n22 = case shown="Error" w85 {
              tunnel: [w99 w100] -> w91
              tunnel: w92 -> [w99 _]
              tunnel: w90 -> [_ w103]
              tunnel: string[] [] -> [_ w102]
              frame No Error {
              }
              frame Error {
                n23 = Variant To Data(type=w102, Variant=w103) -> (data=w101:string[])  [unwired: 1 in, 1 out]
                n24 = Build Array(w101) -> (w100:string[][])
              }
            }
            n25 = Fract/Exp String To Number(string=w91) -> (number=w88:dbl[][])  [unwired: 3 in, 1 out]
            n26 = call "UTILITY DBL Array to String Array.vi"("Error in (no error)"=w85, "Array in"=w88) -> ("Error out"=w84:errorcluster, "String array out"=w87:string)  [unwired: 8 in]
            "String array out" <- w87
            n27 = call-poly <vilib>:"Write Key.vi"("section"=w98, "error in (no error)"=w84, "value"=w87, "key"=w97, "refnum"=w96) -> ("error out"=w95:errorcluster, "refnum out"=w94:T11)  [unwired: 4 in, 1 out]
          }
          frame "Path" {
            n28 = Variant To Data(error in=w105, type=path "C:/" ("configuration file path 2"), Variant=w111) -> (data=w107:path, error out=w104:errorcluster)
            n29 = call-poly <vilib>:"Write Key.vi"("section"=w113, "error in (no error)"=w104, "value"=w107, "key"=w112, "refnum"=w110) -> ("error out"=w109:errorcluster, "refnum out"=w108:T11)  [unwired: 4 in, 1 out]
          }
          frame "Cluster" {
            w129 = refnum<vi> refnum  # Cluster
            n30 = Concatenate Strings(w117, ": " ("string"), w116) -> (w118:string)
            n31 = To More Specific Class(target class=w129, reference=w121, error in=w126) -> (specific class reference=w128:refnum<vi>, error out=w127:errorcluster)
            n32 = property class="Clust"(reference=w128, error in=w127) -> (error out=w114:errorcluster, "Label.Text"=w122:string, "AllObjs[]"=w120:refnum<vi>[])  [unwired: 1 out]
            n33 = for {
              tunnel: w125 -> [_]
              tunnel: w118 -> [w142]
              tunnel: w120 -> [w134] mode=indexing
              tunnel: [w141] -> w124
              tunnel: w122 -> [_]
              tunnel: w119 -> [w137]
              shift-right: [w140] -> w123
              shift-left: w114 -> [w133]
              w139 = refnum<vi> refnum  # Control
              n34 = To More Specific Class(target class=w139, reference=w134, error in=w133) -> (specific class reference=w138:refnum<vi>, error out=w132:errorcluster)
              n35 = property class="Ctl"(reference=w138, error in=w132) -> (error out=w131:errorcluster, "Label.Text"=w130:string, "Value"=w135:variant)  [unwired: 1 out]
              n36 = call <vilib>:"GetTypeInfo.vi"("Variant"=w135) -> ("Type Enum"=w136:T12)  [unwired: 6 in, 4 out]
              n37 = case shown="\"Cluster\"" w136 {
                tunnel: w142 -> [w152 w162 w172 w185 w189 w204 w634 w639 w655 w665 w672 w683]
                tunnel: w130 -> [w151 w161 w165 w184 w188 _ w633 w638 w654 w664 w670 w681]
                tunnel: w135 -> [w150 w160 w171 w183 w195 _ w632 w641 w653 w663 w669 w680]
                tunnel: w137 -> [w145 w155 w166 w178 w190 w205 w626 w637 w647 w658 w671 w682]
                tunnel: [w149 w159 w170 w182 w194 w206 w631 w635 w652 w662 w666 w678] -> w140
                tunnel: [w148 w158 w169 w181 w193 w207 w630 w636 w651 w661 w667 w679] -> w141
                tunnel: w134 -> [_ _ _ _ _ w203 _ _ _ _ _ _]
                tunnel: w131 -> [w144 w154 w164 w175 w187 w199 w625 w640 w646 w657 w668 w677]
                frame "Double Float" {
                  n38 = Variant To Data(error in=w144, type=0.0, Variant=w150) -> (data=w146:dbl, error out=w143:errorcluster)
                  n39 = call-poly <vilib>:"Write Key.vi"("section"=w152, "error in (no error)"=w143, "value"=w146, "key"=w151, "refnum"=w145) -> ("error out"=w149:errorcluster, "refnum out"=w148:T11)  [unwired: 4 in, 1 out]
                }
                frame "String" {
                  n40 = Variant To Data(error in=w154, type="" ("Label.Text"), Variant=w160) -> (data=w156:string, error out=w153:errorcluster)
                  n41 = call-poly <vilib>:"Write Key.vi"("section"=w162, "error in (no error)"=w153, "value"=w156, "key"=w161, "refnum"=w155) -> ("error out"=w159:errorcluster, "refnum out"=w158:T11)  [unwired: 4 in, 1 out]
                }
                frame Default {
                  n42 = Variant To Data(error in=w164, type="" ("Label.Text"), Variant=w171) -> (data=w167:string, error out=w163:errorcluster)
                  n43 = call-poly <vilib>:"Write Key.vi"("section"=w172, "error in (no error)"=w163, "value"=w167, "key"=w165, "refnum"=w166) -> ("error out"=w170:errorcluster, "refnum out"=w169:T11)  [unwired: 4 in, 1 out]
                }
                frame "Array" {
                  n44 = Variant To Data(error in=w175, type=string[][] [], Variant=w183) -> (data=w179:string[][], error out=w174:errorcluster)
                  n45 = Fract/Exp String To Number(string=w179) -> (number=w177:dbl[][])  [unwired: 3 in, 1 out]
                  n46 = call "UTILITY DBL Array to String Array.vi"("Error in (no error)"=w174, "Array in"=w177) -> ("Error out"=w173:errorcluster, "String array out"=w176:string)  [unwired: 8 in]
                  n47 = call-poly <vilib>:"Write Key.vi"("section"=w185, "error in (no error)"=w173, "value"=w176, "key"=w184, "refnum"=w178) -> ("error out"=w182:errorcluster, "refnum out"=w181:T11)  [unwired: 4 in, 1 out]
                }
                frame "Path" {
                  n48 = Variant To Data(error in=w187, type=path "C:/" ("configuration file path 2"), Variant=w195) -> (data=w191:path, error out=w186:errorcluster)
                  n49 = call-poly <vilib>:"Write Key.vi"("section"=w189, "error in (no error)"=w186, "value"=w191, "key"=w188, "refnum"=w190) -> ("error out"=w194:errorcluster, "refnum out"=w193:T11)  [unwired: 4 in, 1 out]
                }
                frame "Cluster" {
                  w202 = refnum<vi> refnum  # Cluster
                  n50 = To More Specific Class(target class=w202, reference=w203, error in=w199) -> (specific class reference=w201:refnum<vi>, error out=w198:errorcluster)
                  n51 = property class="Clust"(reference=w201, error in=w198) -> (error out=w197:errorcluster, "Label.Text"=w196:string, "AllObjs[]"=w200:refnum<vi>[])  [unwired: 1 out]
                  n52 = for {
                    tunnel: w204 -> [w220]
                    tunnel: w200 -> [w212] mode=indexing
                    tunnel: [w219] -> w207
                    tunnel: w205 -> [w217]
                    tunnel: w196 -> [_]
                    shift-right: [w218] -> w206
                    shift-left: w197 -> [w211]
                    w216 = refnum<vi> refnum  # Control
                    n53 = To More Specific Class(target class=w216, reference=w212, error in=w211) -> (specific class reference=w215:refnum<vi>, error out=w210:errorcluster)
                    n54 = property class="Ctl"(reference=w215, error in=w210) -> (error out=w209:errorcluster, "Label.Text"=w208:string, "Value"=w213:variant)  [unwired: 1 out]
                    n55 = call <vilib>:"GetTypeInfo.vi"("Variant"=w213) -> ("Type Enum"=w214:T12)  [unwired: 6 in, 4 out]
                    n56 = case shown="\"Cluster\"" w214 {
                      tunnel: w220 -> [w230 w240 w250 w263 w267 w282 w573 w577 w594 w604 w610 w620]
                      tunnel: w208 -> [w229 w239 w243 w262 w266 _ w572 w578 w593 w603 w608 w621]
                      tunnel: w213 -> [w228 w238 w249 w261 w273 _ w571 w580 w592 w602 w607 w619]
                      tunnel: w217 -> [w223 w233 w244 w256 w268 w281 w565 w576 w586 w597 w609 w622]
                      tunnel: [w227 w237 w248 w260 w272 w279 w570 w574 w591 w601 w612 w617] -> w218
                      tunnel: [w226 w236 w247 w259 w271 w280 w569 w575 w590 w600 w611 w618] -> w219
                      tunnel: w212 -> [_ _ _ _ _ w283 _ _ _ _ _ _]
                      tunnel: w209 -> [w222 w232 w242 w253 w265 w276 w564 w579 w585 w596 w606 w616]
                      frame "Double Float" {
                        n57 = Variant To Data(error in=w222, type=0.0, Variant=w228) -> (data=w224:dbl, error out=w221:errorcluster)
                        n58 = call-poly <vilib>:"Write Key.vi"("section"=w230, "error in (no error)"=w221, "value"=w224, "key"=w229, "refnum"=w223) -> ("error out"=w227:errorcluster, "refnum out"=w226:T11)  [unwired: 4 in, 1 out]
                      }
                      frame "String" {
                        n59 = Variant To Data(error in=w232, type="" ("Label.Text"), Variant=w238) -> (data=w234:string, error out=w231:errorcluster)
                        n60 = call-poly <vilib>:"Write Key.vi"("section"=w240, "error in (no error)"=w231, "value"=w234, "key"=w239, "refnum"=w233) -> ("error out"=w237:errorcluster, "refnum out"=w236:T11)  [unwired: 4 in, 1 out]
                      }
                      frame Default {
                        n61 = Variant To Data(error in=w242, type="" ("Label.Text"), Variant=w249) -> (data=w245:string, error out=w241:errorcluster)
                        n62 = call-poly <vilib>:"Write Key.vi"("section"=w250, "error in (no error)"=w241, "value"=w245, "key"=w243, "refnum"=w244) -> ("error out"=w248:errorcluster, "refnum out"=w247:T11)  [unwired: 4 in, 1 out]
                      }
                      frame "Array" {
                        n63 = Variant To Data(error in=w253, type=string[][] [], Variant=w261) -> (data=w257:string[][], error out=w252:errorcluster)
                        n64 = Fract/Exp String To Number(string=w257) -> (number=w255:dbl[][])  [unwired: 3 in, 1 out]
                        n65 = call "UTILITY DBL Array to String Array.vi"("Error in (no error)"=w252, "Array in"=w255) -> ("Error out"=w251:errorcluster, "String array out"=w254:string)  [unwired: 8 in]
                        n66 = call-poly <vilib>:"Write Key.vi"("section"=w263, "error in (no error)"=w251, "value"=w254, "key"=w262, "refnum"=w256) -> ("error out"=w260:errorcluster, "refnum out"=w259:T11)  [unwired: 4 in, 1 out]
                      }
                      frame "Path" {
                        n67 = Variant To Data(error in=w265, type=path "C:/" ("configuration file path 2"), Variant=w273) -> (data=w269:path, error out=w264:errorcluster)
                        n68 = call-poly <vilib>:"Write Key.vi"("section"=w267, "error in (no error)"=w264, "value"=w269, "key"=w266, "refnum"=w268) -> ("error out"=w272:errorcluster, "refnum out"=w271:T11)  [unwired: 4 in, 1 out]
                      }
                      frame "Cluster" {
                        w284 = refnum<vi> refnum  # Cluster
                        n69 = To More Specific Class(target class=w284, reference=w283, error in=w276) -> (specific class reference=w285:refnum<vi>, error out=w275:errorcluster)
                        n70 = property class="Clust"(reference=w285, error in=w275) -> (error out=w274:errorcluster, "Label.Text"=w278:string, "AllObjs[]"=w277:refnum<vi>[])  [unwired: 1 out]
                        n71 = for {
                          tunnel: w282 -> [w298]
                          tunnel: [w297] -> w280
                          tunnel: w281 -> [w293]
                          tunnel: w277 -> [w289] mode=indexing
                          tunnel: w278 -> [_]
                          shift-right: [w296] -> w279
                          shift-left: w274 -> [w288]
                          w295 = refnum<vi> refnum  # Control
                          n72 = To More Specific Class(target class=w295, reference=w289, error in=w288) -> (specific class reference=w294:refnum<vi>, error out=w287:errorcluster)
                          n73 = property class="Ctl"(reference=w294, error in=w287) -> (error out=w286:errorcluster, "Label.Text"=w290:string, "Value"=w291:variant)  [unwired: 1 out]
                          n74 = call <vilib>:"GetTypeInfo.vi"("Variant"=w291) -> ("Type Enum"=w292:T12)  [unwired: 6 in, 4 out]
                          n75 = case shown="\"Cluster\"" w292 {
                            tunnel: w298 -> [w308 w318 w328 w341 w345 w355 w512 w515 w533 w543 w548 w560]
                            tunnel: w290 -> [w307 w317 w321 w340 w344 _ w511 w517 w532 w542 w546 w558]
                            tunnel: w291 -> [w306 w316 w327 w339 w351 _ w510 w518 w531 w541 w549 w561]
                            tunnel: w293 -> [w301 w311 w322 w334 w346 w356 w504 w516 w525 w536 w547 w559]
                            tunnel: [w305 w315 w326 w338 w350 w362 w509 w513 w530 w540 w544 w556] -> w296
                            tunnel: [w304 w314 w325 w337 w349 w363 w508 w514 w529 w539 w545 w557] -> w297
                            tunnel: w289 -> [_ _ _ _ _ w359 _ _ _ _ _ _]
                            tunnel: w286 -> [w300 w310 w320 w331 w343 w354 w503 w519 w524 w535 w550 w555]
                            frame "Double Float" {
                              n76 = Variant To Data(error in=w300, type=0.0, Variant=w306) -> (data=w302:dbl, error out=w299:errorcluster)
                              n77 = call-poly <vilib>:"Write Key.vi"("section"=w308, "error in (no error)"=w299, "value"=w302, "key"=w307, "refnum"=w301) -> ("error out"=w305:errorcluster, "refnum out"=w304:T11)  [unwired: 4 in, 1 out]
                            }
                            frame "String" {
                              n78 = Variant To Data(error in=w310, type="" ("Label.Text"), Variant=w316) -> (data=w312:string, error out=w309:errorcluster)
                              n79 = call-poly <vilib>:"Write Key.vi"("section"=w318, "error in (no error)"=w309, "value"=w312, "key"=w317, "refnum"=w311) -> ("error out"=w315:errorcluster, "refnum out"=w314:T11)  [unwired: 4 in, 1 out]
                            }
                            frame Default {
                              n80 = Variant To Data(error in=w320, type="" ("Label.Text"), Variant=w327) -> (data=w323:string, error out=w319:errorcluster)
                              n81 = call-poly <vilib>:"Write Key.vi"("section"=w328, "error in (no error)"=w319, "value"=w323, "key"=w321, "refnum"=w322) -> ("error out"=w326:errorcluster, "refnum out"=w325:T11)  [unwired: 4 in, 1 out]
                            }
                            frame "Array" {
                              n82 = Variant To Data(error in=w331, type=string[][] [], Variant=w339) -> (data=w335:string[][], error out=w330:errorcluster)
                              n83 = Fract/Exp String To Number(string=w335) -> (number=w333:dbl[][])  [unwired: 3 in, 1 out]
                              n84 = call "UTILITY DBL Array to String Array.vi"("Error in (no error)"=w330, "Array in"=w333) -> ("Error out"=w329:errorcluster, "String array out"=w332:string)  [unwired: 8 in]
                              n85 = call-poly <vilib>:"Write Key.vi"("section"=w341, "error in (no error)"=w329, "value"=w332, "key"=w340, "refnum"=w334) -> ("error out"=w338:errorcluster, "refnum out"=w337:T11)  [unwired: 4 in, 1 out]
                            }
                            frame "Path" {
                              n86 = Variant To Data(error in=w343, type=path "C:/" ("configuration file path 2"), Variant=w351) -> (data=w347:path, error out=w342:errorcluster)
                              n87 = call-poly <vilib>:"Write Key.vi"("section"=w345, "error in (no error)"=w342, "value"=w347, "key"=w344, "refnum"=w346) -> ("error out"=w350:errorcluster, "refnum out"=w349:T11)  [unwired: 4 in, 1 out]
                            }
                            frame "Cluster" {
                              w361 = refnum<vi> refnum  # Cluster
                              n88 = To More Specific Class(target class=w361, reference=w359, error in=w354) -> (specific class reference=w360:refnum<vi>, error out=w353:errorcluster)
                              n89 = property class="Clust"(reference=w360, error in=w353) -> (error out=w352:errorcluster, "Label.Text"=w357:string, "AllObjs[]"=w358:refnum<vi>[])  [unwired: 1 out]
                              n90 = for {
                                tunnel: w355 -> [w376]
                                tunnel: [w375] -> w363
                                tunnel: w356 -> [w371]
                                tunnel: w358 -> [w367] mode=indexing
                                tunnel: w357 -> [_]
                                shift-right: [w374] -> w362
                                shift-left: w352 -> [w366]
                                w373 = refnum<vi> refnum  # Control
                                n91 = To More Specific Class(target class=w373, reference=w367, error in=w366) -> (specific class reference=w372:refnum<vi>, error out=w365:errorcluster)
                                n92 = property class="Ctl"(reference=w372, error in=w365) -> (error out=w364:errorcluster, "Label.Text"=w368:string, "Value"=w369:variant)  [unwired: 1 out]
                                n93 = call <vilib>:"GetTypeInfo.vi"("Variant"=w369) -> ("Type Enum"=w370:T12)  [unwired: 6 in, 4 out]
                                n94 = case shown="Default" w370 {
                                tunnel: w376 -> [w386 w396 w406 w419 w423 w434 w451 w453 w472 w482 w487 w500]
                                tunnel: w368 -> [w385 w395 w399 w418 w422 _ w450 w452 w471 w481 w485 w498]
                                tunnel: w369 -> [w384 w394 w405 w417 w429 _ w449 w455 w470 w480 w488 w497]
                                tunnel: w371 -> [w379 w389 w400 w412 w424 w433 w443 w454 w464 w475 w486 w499]
                                tunnel: [w383 w393 w404 w416 w428 w440 w448 w457 w469 w479 w483 w495] -> w374
                                tunnel: [w382 w392 w403 w415 w427 w441 w447 w458 w468 w478 w484 w496] -> w375
                                tunnel: w367 -> [_ _ _ _ _ w437 _ _ _ _ _ _]
                                tunnel: w364 -> [w378 w388 w398 w409 w421 w432 w442 w456 w463 w474 w489 w494]
                                frame "Double Float" {
                                n95 = Variant To Data(error in=w378, type=0.0, Variant=w384) -> (data=w380:dbl, error out=w377:errorcluster)
                                n96 = call-poly <vilib>:"Write Key.vi"("section"=w386, "error in (no error)"=w377, "value"=w380, "key"=w385, "refnum"=w379) -> ("error out"=w383:errorcluster, "refnum out"=w382:T11)  [unwired: 4 in, 1 out]
                                }
                                frame "String" {
                                n97 = Variant To Data(error in=w388, type="" ("Label.Text"), Variant=w394) -> (data=w390:string, error out=w387:errorcluster)
                                n98 = call-poly <vilib>:"Write Key.vi"("section"=w396, "error in (no error)"=w387, "value"=w390, "key"=w395, "refnum"=w389) -> ("error out"=w393:errorcluster, "refnum out"=w392:T11)  [unwired: 4 in, 1 out]
                                }
                                frame Default {
                                n99 = Variant To Data(error in=w398, type="" ("Label.Text"), Variant=w405) -> (data=w401:string, error out=w397:errorcluster)
                                n100 = call-poly <vilib>:"Write Key.vi"("section"=w406, "error in (no error)"=w397, "value"=w401, "key"=w399, "refnum"=w400) -> ("error out"=w404:errorcluster, "refnum out"=w403:T11)  [unwired: 4 in, 1 out]
                                }
                                frame "Array" {
                                n101 = Variant To Data(error in=w409, type=string[][] [], Variant=w417) -> (data=w413:string[][], error out=w408:errorcluster)
                                n102 = Fract/Exp String To Number(string=w413) -> (number=w411:dbl[][])  [unwired: 3 in, 1 out]
                                n103 = call "UTILITY DBL Array to String Array.vi"("Error in (no error)"=w408, "Array in"=w411) -> ("Error out"=w407:errorcluster, "String array out"=w410:string)  [unwired: 8 in]
                                n104 = call-poly <vilib>:"Write Key.vi"("section"=w419, "error in (no error)"=w407, "value"=w410, "key"=w418, "refnum"=w412) -> ("error out"=w416:errorcluster, "refnum out"=w415:T11)  [unwired: 4 in, 1 out]
                                }
                                frame "Path" {
                                n105 = Variant To Data(error in=w421, type=path "C:/" ("configuration file path 2"), Variant=w429) -> (data=w425:path, error out=w420:errorcluster)
                                n106 = call-poly <vilib>:"Write Key.vi"("section"=w423, "error in (no error)"=w420, "value"=w425, "key"=w422, "refnum"=w424) -> ("error out"=w428:errorcluster, "refnum out"=w427:T11)  [unwired: 4 in, 1 out]
                                }
                                frame "Cluster" {
                                w438 = refnum<vi> refnum  # Cluster
                                n107 = To More Specific Class(target class=w438, reference=w437, error in=w432) -> (specific class reference=w439:refnum<vi>, error out=w431:errorcluster)
                                n108 = property class="Clust"(reference=w439, error in=w431) -> (error out=w430:errorcluster, "Label.Text"=w436:string, "AllObjs[]"=w435:refnum<vi>[])  [unwired: 1 out]
                                n109 = call "Final_Write_Key.vi"("AllObjs[]"=w435, "error in (no error)"=w430, "Label.Text"=w436, "String"=w434, "Refnum in"=w433) -> ("error out"=w440:errorcluster, "Refnum out"=w441:T11)  [unwired: 5 in]
                                }
                                frame "I32" {
                                n110 = Variant To Data(error in=w442, type=0, Variant=w449) -> (data=w444:i32, error out=w445:errorcluster)
                                n111 = call-poly <vilib>:"Write Key.vi"("section"=w451, "error in (no error)"=w445, "value"=w444, "key"=w450, "refnum"=w443) -> ("error out"=w448:errorcluster, "refnum out"=w447:T11)  [unwired: 4 in, 1 out]
                                }
                                frame "U32" {
                                n112 = Variant To Data(error in=w456, type=0, Variant=w455) -> (data=w461:i32, error out=w459:errorcluster)
                                n113 = call-poly <vilib>:"Write Key.vi"("section"=w453, "error in (no error)"=w459, "value"=w461, "key"=w452, "refnum"=w454) -> ("error out"=w457:errorcluster, "refnum out"=w458:T11)  [unwired: 4 in, 1 out]
                                }
                                frame "U8" {
                                n114 = Variant To Data(error in=w463, type=u8 0, Variant=w470) -> (data=w467:u8, error out=w462:errorcluster)
                                n115 = To Unsigned Long Integer(number=w467) -> (unsigned 32bit integer=w465:u32)
                                n116 = call-poly <vilib>:"Write Key.vi"("section"=w472, "error in (no error)"=w462, "value"=w465, "key"=w471, "refnum"=w464) -> ("error out"=w469:errorcluster, "refnum out"=w468:T11)  [unwired: 4 in, 1 out]
                                }
                                frame "Boolean" {
                                n117 = Variant To Data(error in=w474, type=FALSE ("Write? 2"), Variant=w480) -> (data=w477:bool, error out=w473:errorcluster)
                                n118 = call-poly <vilib>:"Write Key.vi"("section"=w482, "error in (no error)"=w473, "value"=w477, "key"=w481, "refnum"=w475) -> ("error out"=w479:errorcluster, "refnum out"=w478:T11)  [unwired: 4 in, 1 out]
                                }
                                frame "Enum U8" {
                                n119 = Variant To Data(error in=w489, type=enum32{""}."" ("Enum"), Variant=w488) -> (data=w492:enum32{""}, error out=w490:errorcluster)
                                n120 = call-poly <vilib>:"Write Key.vi"("section"=w487, "error in (no error)"=w490, "value"=w492, "key"=w485, "refnum"=w486) -> ("error out"=w483:errorcluster, "refnum out"=w484:T11)  [unwired: 4 in, 1 out]
                                }
                                frame "Refnum" {
                                n121 = Variant To Data(error in=w494, type=refnum<visa-resource-name> refnum ("VISA resource name"), Variant=w497) -> (data=w502:refnum<visa-resource-name>, error out=w493:errorcluster)
                                n122 = call-poly <vilib>:"Write Key.vi"("section"=w500, "error in (no error)"=w493, "value"=w502, "key"=w498, "refnum"=w499) -> ("error out"=w495:errorcluster, "refnum out"=w496:T11)  [unwired: 4 in, 1 out]
                                }
                                }
                              }
                            }
                            frame "I32" {
                              n123 = Variant To Data(error in=w503, type=0, Variant=w510) -> (data=w505:i32, error out=w506:errorcluster)
                              n124 = call-poly <vilib>:"Write Key.vi"("section"=w512, "error in (no error)"=w506, "value"=w505, "key"=w511, "refnum"=w504) -> ("error out"=w509:errorcluster, "refnum out"=w508:T11)  [unwired: 4 in, 1 out]
                            }
                            frame "U32" {
                              n125 = Variant To Data(error in=w519, type=0, Variant=w518) -> (data=w522:i32, error out=w520:errorcluster)
                              n126 = call-poly <vilib>:"Write Key.vi"("section"=w515, "error in (no error)"=w520, "value"=w522, "key"=w517, "refnum"=w516) -> ("error out"=w513:errorcluster, "refnum out"=w514:T11)  [unwired: 4 in, 1 out]
                            }
                            frame "U8" {
                              n127 = Variant To Data(error in=w524, type=u8 0, Variant=w531) -> (data=w528:u8, error out=w523:errorcluster)
                              n128 = To Unsigned Long Integer(number=w528) -> (unsigned 32bit integer=w526:u32)
                              n129 = call-poly <vilib>:"Write Key.vi"("section"=w533, "error in (no error)"=w523, "value"=w526, "key"=w532, "refnum"=w525) -> ("error out"=w530:errorcluster, "refnum out"=w529:T11)  [unwired: 4 in, 1 out]
                            }
                            frame "Boolean" {
                              n130 = Variant To Data(error in=w535, type=FALSE ("Write? 2"), Variant=w541) -> (data=w538:bool, error out=w534:errorcluster)
                              n131 = call-poly <vilib>:"Write Key.vi"("section"=w543, "error in (no error)"=w534, "value"=w538, "key"=w542, "refnum"=w536) -> ("error out"=w540:errorcluster, "refnum out"=w539:T11)  [unwired: 4 in, 1 out]
                            }
                            frame "Enum U8" {
                              n132 = Variant To Data(error in=w550, type=enum32{""}."" ("Enum"), Variant=w549) -> (data=w553:enum32{""}, error out=w551:errorcluster)
                              n133 = call-poly <vilib>:"Write Key.vi"("section"=w548, "error in (no error)"=w551, "value"=w553, "key"=w546, "refnum"=w547) -> ("error out"=w544:errorcluster, "refnum out"=w545:T11)  [unwired: 4 in, 1 out]
                            }
                            frame "Refnum" {
                              n134 = Variant To Data(error in=w555, type=refnum<visa-resource-name> refnum ("VISA resource name"), Variant=w561) -> (data=w563:refnum<visa-resource-name>, error out=w554:errorcluster)
                              n135 = call-poly <vilib>:"Write Key.vi"("section"=w560, "error in (no error)"=w554, "value"=w563, "key"=w558, "refnum"=w559) -> ("error out"=w556:errorcluster, "refnum out"=w557:T11)  [unwired: 4 in, 1 out]
                            }
                          }
                        }
                      }
                      frame "I32" {
                        n136 = Variant To Data(error in=w564, type=0, Variant=w571) -> (data=w566:i32, error out=w567:errorcluster)
                        n137 = call-poly <vilib>:"Write Key.vi"("section"=w573, "error in (no error)"=w567, "value"=w566, "key"=w572, "refnum"=w565) -> ("error out"=w570:errorcluster, "refnum out"=w569:T11)  [unwired: 4 in, 1 out]
                      }
                      frame "U32" {
                        n138 = Variant To Data(error in=w579, type=0, Variant=w580) -> (data=w583:i32, error out=w581:errorcluster)
                        n139 = call-poly <vilib>:"Write Key.vi"("section"=w577, "error in (no error)"=w581, "value"=w583, "key"=w578, "refnum"=w576) -> ("error out"=w574:errorcluster, "refnum out"=w575:T11)  [unwired: 4 in, 1 out]
                      }
                      frame "U8" {
                        n140 = Variant To Data(error in=w585, type=u8 0, Variant=w592) -> (data=w589:u8, error out=w584:errorcluster)
                        n141 = To Unsigned Long Integer(number=w589) -> (unsigned 32bit integer=w587:u32)
                        n142 = call-poly <vilib>:"Write Key.vi"("section"=w594, "error in (no error)"=w584, "value"=w587, "key"=w593, "refnum"=w586) -> ("error out"=w591:errorcluster, "refnum out"=w590:T11)  [unwired: 4 in, 1 out]
                      }
                      frame "Boolean" {
                        n143 = Variant To Data(error in=w596, type=FALSE ("Write? 2"), Variant=w602) -> (data=w599:bool, error out=w595:errorcluster)
                        n144 = call-poly <vilib>:"Write Key.vi"("section"=w604, "error in (no error)"=w595, "value"=w599, "key"=w603, "refnum"=w597) -> ("error out"=w601:errorcluster, "refnum out"=w600:T11)  [unwired: 4 in, 1 out]
                      }
                      frame "Enum U8" {
                        n145 = Variant To Data(error in=w606, type=enum32{""}."" ("Enum"), Variant=w607) -> (data=w614:enum32{""}, error out=w605:errorcluster)
                        n146 = call-poly <vilib>:"Write Key.vi"("section"=w610, "error in (no error)"=w605, "value"=w614, "key"=w608, "refnum"=w609) -> ("error out"=w612:errorcluster, "refnum out"=w611:T11)  [unwired: 4 in, 1 out]
                      }
                      frame "Refnum" {
                        n147 = Variant To Data(error in=w616, type=refnum<visa-resource-name> refnum ("VISA resource name"), Variant=w619) -> (data=w624:refnum<visa-resource-name>, error out=w615:errorcluster)
                        n148 = call-poly <vilib>:"Write Key.vi"("section"=w620, "error in (no error)"=w615, "value"=w624, "key"=w621, "refnum"=w622) -> ("error out"=w617:errorcluster, "refnum out"=w618:T11)  [unwired: 4 in, 1 out]
                      }
                    }
                  }
                }
                frame "I32" {
                  n149 = Variant To Data(error in=w625, type=0, Variant=w632) -> (data=w627:i32, error out=w628:errorcluster)
                  n150 = call-poly <vilib>:"Write Key.vi"("section"=w634, "error in (no error)"=w628, "value"=w627, "key"=w633, "refnum"=w626) -> ("error out"=w631:errorcluster, "refnum out"=w630:T11)  [unwired: 4 in, 1 out]
                }
                frame "U32" {
                  n151 = Variant To Data(error in=w640, type=0, Variant=w641) -> (data=w644:i32, error out=w642:errorcluster)
                  n152 = call-poly <vilib>:"Write Key.vi"("section"=w639, "error in (no error)"=w642, "value"=w644, "key"=w638, "refnum"=w637) -> ("error out"=w635:errorcluster, "refnum out"=w636:T11)  [unwired: 4 in, 1 out]
                }
                frame "U8" {
                  n153 = Variant To Data(error in=w646, type=u8 0, Variant=w653) -> (data=w650:u8, error out=w645:errorcluster)
                  n154 = To Unsigned Long Integer(number=w650) -> (unsigned 32bit integer=w648:u32)
                  n155 = call-poly <vilib>:"Write Key.vi"("section"=w655, "error in (no error)"=w645, "value"=w648, "key"=w654, "refnum"=w647) -> ("error out"=w652:errorcluster, "refnum out"=w651:T11)  [unwired: 4 in, 1 out]
                }
                frame "Boolean" {
                  n156 = Variant To Data(error in=w657, type=FALSE ("Write? 2"), Variant=w663) -> (data=w660:bool, error out=w656:errorcluster)
                  n157 = call-poly <vilib>:"Write Key.vi"("section"=w665, "error in (no error)"=w656, "value"=w660, "key"=w664, "refnum"=w658) -> ("error out"=w662:errorcluster, "refnum out"=w661:T11)  [unwired: 4 in, 1 out]
                }
                frame "Enum U8" {
                  n158 = Variant To Data(error in=w668, type=enum32{""}."" ("Enum"), Variant=w669) -> (data=w675:enum32{""}, error out=w673:errorcluster)
                  n159 = call-poly <vilib>:"Write Key.vi"("section"=w672, "error in (no error)"=w673, "value"=w675, "key"=w670, "refnum"=w671) -> ("error out"=w666:errorcluster, "refnum out"=w667:T11)  [unwired: 4 in, 1 out]
                }
                frame "Refnum" {
                  n160 = Variant To Data(error in=w677, type=refnum<visa-resource-name> refnum ("VISA resource name"), Variant=w680) -> (data=w685:refnum<visa-resource-name>, error out=w676:errorcluster)
                  n161 = call-poly <vilib>:"Write Key.vi"("section"=w683, "error in (no error)"=w676, "value"=w685, "key"=w681, "refnum"=w682) -> ("error out"=w678:errorcluster, "refnum out"=w679:T11)  [unwired: 4 in, 1 out]
                }
              }
            }
          }
          frame "I32" {
            n162 = Variant To Data(error in=w687, type=0, Variant=w693) -> (data=w689:i32, error out=w686:errorcluster)
            n163 = call-poly <vilib>:"Write Key.vi"("section"=w695, "error in (no error)"=w686, "value"=w689, "key"=w694, "refnum"=w692) -> ("error out"=w691:errorcluster, "refnum out"=w690:T11)  [unwired: 4 in, 1 out]
          }
          frame "U32" {
            n164 = Variant To Data(error in=w697, type=0, Variant=w703) -> (data=w699:i32, error out=w696:errorcluster)
            n165 = call-poly <vilib>:"Write Key.vi"("section"=w705, "error in (no error)"=w696, "value"=w699, "key"=w704, "refnum"=w702) -> ("error out"=w701:errorcluster, "refnum out"=w700:T11)  [unwired: 4 in, 1 out]
          }
          frame "U8" {
            n166 = Variant To Data(error in=w707, type=u8 0, Variant=w714) -> (data=w710:u8, error out=w706:errorcluster)
            n167 = To Unsigned Long Integer(number=w710) -> (unsigned 32bit integer=w708:u32)
            n168 = call-poly <vilib>:"Write Key.vi"("section"=w716, "error in (no error)"=w706, "value"=w708, "key"=w715, "refnum"=w713) -> ("error out"=w712:errorcluster, "refnum out"=w711:T11)  [unwired: 4 in, 1 out]
          }
          frame "Boolean" {
            n169 = Variant To Data(error in=w718, type=FALSE ("Write? 2"), Variant=w724) -> (data=w720:bool, error out=w717:errorcluster)
            n170 = call-poly <vilib>:"Write Key.vi"("section"=w726, "error in (no error)"=w717, "value"=w720, "key"=w725, "refnum"=w723) -> ("error out"=w722:errorcluster, "refnum out"=w721:T11)  [unwired: 4 in, 1 out]
          }
          frame "Enum U8" {
            n171 = Variant To Data(error in=w728, type=enum32{""}."" ("Enum"), Variant=w733) -> (data=w736:enum32{""}, error out=w727:errorcluster)
            n172 = call-poly <vilib>:"Write Key.vi"("section"=w734, "error in (no error)"=w727, "value"=w736, "key"=w731, "refnum"=w732) -> ("error out"=w729:errorcluster, "refnum out"=w730:T11)  [unwired: 4 in, 1 out]
          }
          frame "Refnum" {
            n173 = Variant To Data(error in=w738, type=refnum<visa-resource-name> refnum ("VISA resource name"), Variant=w741) -> (data=w746:refnum<visa-resource-name>, error out=w737:errorcluster)
            n174 = call-poly <vilib>:"Write Key.vi"("section"=w744, "error in (no error)"=w737, "value"=w746, "key"=w742, "refnum"=w743) -> ("error out"=w739:errorcluster, "refnum out"=w740:T11)  [unwired: 4 in, 1 out]
          }
        }
      }
      frame False {
        n175 = case shown="\"Enum U8\"" w747 {
          tunnel: w755 -> [w762 w770 w778 w786 w795 w801 w1162 w1170 w1178 w1186 w1194 w1202]
          tunnel: w754 -> [w761 w769 w777 w783 w794 w800 w1161 w1169 w1176 w1184 w1192 w1201]
          tunnel: w752 -> [_ _ _ _ _ w808 _ _ _ _ _ _]
          tunnel: w751 -> [w760 w768 w776 w784 w793 w803 w1160 w1168 w1177 w1185 w1193 w1200]
          tunnel: [w757 w765 w773 w781 w790 w806 w1158 w1165 w1173 w1181 w1189 w1197] -> w748
          tunnel: [w758 w766 w774 w782 w791 w807 w1157 w1166 w1174 w1182 w1190 w1198] -> w749
          tunnel: w753 -> [w756 w764 w772 w780 w789 w809 w1156 w1164 w1172 w1180 w1188 w1196]
          tunnel: w750 -> [w759 w767 w775 w785 w792 w805 w1159 w1167 w1175 w1183 w1191 w1199]
          frame "Double Float" {
            n176 = call-poly <vilib>:"Read Key.vi"("section"=w762, "error in (no error)"=w756, "key"=w761, "refnum"=w760) -> ("error out"=w757:errorcluster, "value"=w763:dbl, "refnum out"=w758:T11)  [unwired: 4 in, 1 out]
            n177 = property class="Ctl"(reference=w759, "Value"=w763) -> ()  [unwired: 1 in, 2 out]
          }
          frame "String" {
            n178 = call-poly <vilib>:"Read Key.vi"("section"=w770, "error in (no error)"=w764, "key"=w769, "refnum"=w768) -> ("error out"=w765:errorcluster, "value"=w771:string, "refnum out"=w766:T11)  [unwired: 4 in, 1 out]
            n179 = property class="Ctl"(reference=w767, "Value"=w771) -> ()  [unwired: 1 in, 2 out]
          }
          frame Default {
            n180 = call-poly <vilib>:"Read Key.vi"("section"=w778, "error in (no error)"=w772, "key"=w777, "refnum"=w776) -> ("error out"=w773:errorcluster, "value"=w779:string, "refnum out"=w774:T11)  [unwired: 4 in, 1 out]
            n181 = property class="Ctl"(reference=w775, "Value"=w779) -> ()  [unwired: 1 in, 2 out]
          }
          frame "Array" {
            n182 = call-poly <vilib>:"Read Key.vi"("section"=w786, "error in (no error)"=w780, "key"=w783, "refnum"=w784) -> ("error out"=w781:errorcluster, "value"=w787:string, "refnum out"=w782:T11)  [unwired: 4 in, 1 out]
            n183 = call "UTILITY String Array to DBL Array.vi"("String array in"=w787) -> ("Double array out"=w788:dbl[][])  [unwired: 9 in, 1 out]
            n184 = property class="Ctl"(reference=w785, "Value"=w788) -> ()  [unwired: 1 in, 2 out]
          }
          frame "Path" {
            n185 = call-poly <vilib>:"Read Key.vi"("section"=w795, "error in (no error)"=w789, "key"=w794, "refnum"=w793) -> ("error out"=w790:errorcluster, "value"=w796:path, "refnum out"=w791:T11)  [unwired: 4 in, 1 out]
            n186 = property class="Ctl"(reference=w792, "Value"=w796) -> ()  [unwired: 1 in, 2 out]
          }
          frame "Cluster" {
            w812 = refnum<vi> refnum  # Cluster
            n187 = Concatenate Strings(w801, ": " ("string"), w800) -> (w802:string)
            n188 = To More Specific Class(target class=w812, reference=w805, error in=w809) -> (specific class reference=w811:refnum<vi>, error out=w810:errorcluster)
            n189 = property class="Clust"(reference=w811, error in=w810) -> (error out=w798:errorcluster, "Label.Text"=w797:string, "AllObjs[]"=w804:refnum<vi>[])  [unwired: 1 out]
            n190 = for {
              tunnel: w808 -> [_]
              tunnel: w802 -> [w826]
              tunnel: w804 -> [w817] mode=indexing
              tunnel: [w825] -> w807
              tunnel: w797 -> [_]
              tunnel: w803 -> [w821]
              shift-right: [w824] -> w806
              shift-left: w798 -> [w815]
              w823 = refnum<vi> refnum  # Control
              n191 = To More Specific Class(target class=w823, reference=w817, error in=w815) -> (specific class reference=w822:refnum<vi>, error out=w814:errorcluster)
              n192 = property class="Ctl"(reference=w822, error in=w814) -> (reference out=w816:refnum<vi>, error out=w813:errorcluster, "Label.Text"=w818:string, "Value"=w819:variant)
              n193 = call <vilib>:"GetTypeInfo.vi"("Variant"=w819) -> ("Type Enum"=w820:T12)  [unwired: 6 in, 4 out]
              n194 = case shown="\"Enum U8\"" w820 {
                tunnel: w826 -> [w833 w841 w849 w857 w866 w876 w1114 w1122 w1130 w1138 w1146 w1154]
                tunnel: w818 -> [w831 w839 w848 w852 w864 _ w1113 w1120 w1129 w1137 w1144 w1153]
                tunnel: w819 -> [_ _ _ _ _ _ _ _ _ _ _ _]
                tunnel: w821 -> [w832 w836 w844 w853 w863 w877 w1112 w1121 w1127 w1135 w1145 w1152]
                tunnel: [w828 w837 w845 w854 w861 w878 w1109 w1117 w1125 w1133 w1141 w1149] -> w824
                tunnel: [w829 w838 w846 w855 w862 w879 w1110 w1118 w1126 w1134 w1142 w1150] -> w825
                tunnel: w816 -> [w834 w840 w847 w856 w865 w875 w1111 w1119 w1128 w1136 w1143 w1151]
                tunnel: w813 -> [w827 w835 w843 w851 w860 w870 w1108 w1116 w1124 w1132 w1140 w1148]
                frame "Double Float" {
                  n195 = call-poly <vilib>:"Read Key.vi"("section"=w833, "error in (no error)"=w827, "key"=w831, "refnum"=w832) -> ("error out"=w828:errorcluster, "value"=w830:dbl, "refnum out"=w829:T11)  [unwired: 4 in, 1 out]
                  n196 = property class="Ctl"(reference=w834, "Value"=w830) -> ()  [unwired: 1 in, 2 out]
                }
                frame "String" {
                  n197 = call-poly <vilib>:"Read Key.vi"("section"=w841, "error in (no error)"=w835, "key"=w839, "refnum"=w836) -> ("error out"=w837:errorcluster, "value"=w842:string, "refnum out"=w838:T11)  [unwired: 4 in, 1 out]
                  n198 = property class="Ctl"(reference=w840, "Value"=w842) -> ()  [unwired: 1 in, 2 out]
                }
                frame Default {
                  n199 = call-poly <vilib>:"Read Key.vi"("section"=w849, "error in (no error)"=w843, "key"=w848, "refnum"=w844) -> ("error out"=w845:errorcluster, "value"=w850:string, "refnum out"=w846:T11)  [unwired: 4 in, 1 out]
                  n200 = property class="Ctl"(reference=w847, "Value"=w850) -> ()  [unwired: 1 in, 2 out]
                }
                frame "Array" {
                  n201 = call-poly <vilib>:"Read Key.vi"("section"=w857, "error in (no error)"=w851, "key"=w852, "refnum"=w853) -> ("error out"=w854:errorcluster, "value"=w858:string, "refnum out"=w855:T11)  [unwired: 4 in, 1 out]
                  n202 = call "UTILITY String Array to DBL Array.vi"("String array in"=w858) -> ("Double array out"=w859:dbl[][])  [unwired: 9 in, 1 out]
                  n203 = property class="Ctl"(reference=w856, "Value"=w859) -> ()  [unwired: 1 in, 2 out]
                }
                frame "Path" {
                  n204 = call-poly <vilib>:"Read Key.vi"("section"=w866, "error in (no error)"=w860, "key"=w864, "refnum"=w863) -> ("error out"=w861:errorcluster, "value"=w867:path, "refnum out"=w862:T11)  [unwired: 4 in, 1 out]
                  n205 = property class="Ctl"(reference=w865, "Value"=w867) -> ()  [unwired: 1 in, 2 out]
                }
                frame "Cluster" {
                  w874 = refnum<vi> refnum  # Cluster
                  n206 = To More Specific Class(target class=w874, reference=w875, error in=w870) -> (specific class reference=w873:refnum<vi>, error out=w869:errorcluster)
                  n207 = property class="Clust"(reference=w873, error in=w869) -> (error out=w868:errorcluster, "Label.Text"=w871:string, "AllObjs[]"=w872:refnum<vi>[])  [unwired: 1 out]
                  n208 = for {
                    tunnel: w876 -> [w893]
                    tunnel: w872 -> [w885] mode=indexing
                    tunnel: [w892] -> w879
                    tunnel: w877 -> [w890]
                    tunnel: w871 -> [_]
                    shift-right: [w891] -> w878
                    shift-left: w868 -> [w882]
                    w889 = refnum<vi> refnum  # Control
                    n209 = To More Specific Class(target class=w889, reference=w885, error in=w882) -> (specific class reference=w888:refnum<vi>, error out=w881:errorcluster)
                    n210 = property class="Ctl"(reference=w888, error in=w881) -> (reference out=w884:refnum<vi>, error out=w880:errorcluster, "Label.Text"=w883:string, "Value"=w886:variant)
                    n211 = call <vilib>:"GetTypeInfo.vi"("Variant"=w886) -> ("Type Enum"=w887:T12)  [unwired: 6 in, 4 out]
                    n212 = case shown="\"Enum U8\"" w887 {
                      tunnel: w893 -> [w900 w908 w916 w924 w933 w941 w1066 w1074 w1082 w1090 w1098 w1106]
                      tunnel: w883 -> [w899 w907 w915 w921 w932 _ w1065 w1072 w1081 w1089 w1096 w1105]
                      tunnel: w886 -> [_ _ _ _ _ _ _ _ _ _ _ _]
                      tunnel: w890 -> [w898 w905 w913 w922 w931 w940 w1064 w1073 w1080 w1088 w1097 w1104]
                      tunnel: [w895 w903 w911 w919 w928 w938 w1061 w1069 w1077 w1085 w1093 w1101] -> w891
                      tunnel: [w896 w904 w912 w920 w929 w939 w1062 w1070 w1078 w1086 w1094 w1102] -> w892
                      tunnel: w884 -> [w897 w906 w914 w923 w930 w942 w1063 w1071 w1079 w1087 w1095 w1103]
                      tunnel: w880 -> [w894 w902 w910 w918 w927 w935 w1060 w1068 w1076 w1084 w1092 w1100]
                      frame "Double Float" {
                        n213 = call-poly <vilib>:"Read Key.vi"("section"=w900, "error in (no error)"=w894, "key"=w899, "refnum"=w898) -> ("error out"=w895:errorcluster, "value"=w901:dbl, "refnum out"=w896:T11)  [unwired: 4 in, 1 out]
                        n214 = property class="Ctl"(reference=w897, "Value"=w901) -> ()  [unwired: 1 in, 2 out]
                      }
                      frame "String" {
                        n215 = call-poly <vilib>:"Read Key.vi"("section"=w908, "error in (no error)"=w902, "key"=w907, "refnum"=w905) -> ("error out"=w903:errorcluster, "value"=w909:string, "refnum out"=w904:T11)  [unwired: 4 in, 1 out]
                        n216 = property class="Ctl"(reference=w906, "Value"=w909) -> ()  [unwired: 1 in, 2 out]
                      }
                      frame Default {
                        n217 = call-poly <vilib>:"Read Key.vi"("section"=w916, "error in (no error)"=w910, "key"=w915, "refnum"=w913) -> ("error out"=w911:errorcluster, "value"=w917:string, "refnum out"=w912:T11)  [unwired: 4 in, 1 out]
                        n218 = property class="Ctl"(reference=w914, "Value"=w917) -> ()  [unwired: 1 in, 2 out]
                      }
                      frame "Array" {
                        n219 = call-poly <vilib>:"Read Key.vi"("section"=w924, "error in (no error)"=w918, "key"=w921, "refnum"=w922) -> ("error out"=w919:errorcluster, "value"=w925:string, "refnum out"=w920:T11)  [unwired: 4 in, 1 out]
                        n220 = call "UTILITY String Array to DBL Array.vi"("String array in"=w925) -> ("Double array out"=w926:dbl[][])  [unwired: 9 in, 1 out]
                        n221 = property class="Ctl"(reference=w923, "Value"=w926) -> ()  [unwired: 1 in, 2 out]
                      }
                      frame "Path" {
                        n222 = call-poly <vilib>:"Read Key.vi"("section"=w933, "error in (no error)"=w927, "key"=w932, "refnum"=w931) -> ("error out"=w928:errorcluster, "value"=w934:path, "refnum out"=w929:T11)  [unwired: 4 in, 1 out]
                        n223 = property class="Ctl"(reference=w930, "Value"=w934) -> ()  [unwired: 1 in, 2 out]
                      }
                      frame "Cluster" {
                        w943 = refnum<vi> refnum  # Cluster
                        n224 = To More Specific Class(target class=w943, reference=w942) -> (specific class reference=w944:refnum<vi>)  [unwired: 1 in, 1 out]
                        n225 = property class="Clust"(reference=w944) -> ("Label.Text"=w937:string, "AllObjs[]"=w936:refnum<vi>[])  [unwired: 1 in, 2 out]
                        n226 = for {
                          tunnel: w941 -> [w958]
                          tunnel: [w957] -> w939
                          tunnel: w940 -> [w953]
                          tunnel: w936 -> [w949] mode=indexing
                          tunnel: w937 -> [_]
                          shift-right: [w956] -> w938
                          shift-left: w935 -> [w947]
                          w955 = refnum<vi> refnum  # Control
                          n227 = To More Specific Class(target class=w955, reference=w949, error in=w947) -> (specific class reference=w954:refnum<vi>, error out=w946:errorcluster)
                          n228 = property class="Ctl"(reference=w954, error in=w946) -> (reference out=w948:refnum<vi>, error out=w945:errorcluster, "Label.Text"=w950:string, "Value"=w951:variant)
                          n229 = call <vilib>:"GetTypeInfo.vi"("Variant"=w951) -> ("Type Enum"=w952:T12)  [unwired: 6 in, 4 out]
                          n230 = case shown="\"Cluster\"" w952 {
                            tunnel: w958 -> [w964 w973 w981 w989 w998 w1003 w1018 w1026 w1034 w1042 w1050 w1058]
                            tunnel: w950 -> [w963 w970 w980 w987 w997 _ w1017 w1024 w1032 w1041 w1048 w1057]
                            tunnel: w951 -> [_ _ _ _ _ _ _ _ _ _ _ _]
                            tunnel: w953 -> [w965 w972 w979 w988 w995 w1004 w1016 w1025 w1033 w1040 w1049 w1056]
                            tunnel: [w960 w968 w976 w984 w993 w1010 w1013 w1021 w1029 w1037 w1045 w1053] -> w956
                            tunnel: [w961 w969 w977 w985 w994 w1011 w1014 w1022 w1030 w1038 w1046 w1054] -> w957
                            tunnel: w948 -> [w962 w971 w978 w986 w996 w1007 w1015 w1023 w1031 w1039 w1047 w1055]
                            tunnel: w945 -> [w959 w967 w975 w983 w992 w1002 w1012 w1020 w1028 w1036 w1044 w1052]
                            frame "Double Float" {
                              n231 = call-poly <vilib>:"Read Key.vi"("section"=w964, "error in (no error)"=w959, "key"=w963, "refnum"=w965) -> ("error out"=w960:errorcluster, "value"=w966:dbl, "refnum out"=w961:T11)  [unwired: 4 in, 1 out]
                              n232 = property class="Ctl"(reference=w962, "Value"=w966) -> ()  [unwired: 1 in, 2 out]
                            }
                            frame "String" {
                              n233 = call-poly <vilib>:"Read Key.vi"("section"=w973, "error in (no error)"=w967, "key"=w970, "refnum"=w972) -> ("error out"=w968:errorcluster, "value"=w974:string, "refnum out"=w969:T11)  [unwired: 4 in, 1 out]
                              n234 = property class="Ctl"(reference=w971, "Value"=w974) -> ()  [unwired: 1 in, 2 out]
                            }
                            frame Default {
                              n235 = call-poly <vilib>:"Read Key.vi"("section"=w981, "error in (no error)"=w975, "key"=w980, "refnum"=w979) -> ("error out"=w976:errorcluster, "value"=w982:string, "refnum out"=w977:T11)  [unwired: 4 in, 1 out]
                              n236 = property class="Ctl"(reference=w978, "Value"=w982) -> ()  [unwired: 1 in, 2 out]
                            }
                            frame "Array" {
                              n237 = call-poly <vilib>:"Read Key.vi"("section"=w989, "error in (no error)"=w983, "key"=w987, "refnum"=w988) -> ("error out"=w984:errorcluster, "value"=w990:string, "refnum out"=w985:T11)  [unwired: 4 in, 1 out]
                              n238 = call "UTILITY String Array to DBL Array.vi"("String array in"=w990) -> ("Double array out"=w991:dbl[][])  [unwired: 9 in, 1 out]
                              n239 = property class="Ctl"(reference=w986, "Value"=w991) -> ()  [unwired: 1 in, 2 out]
                            }
                            frame "Path" {
                              n240 = call-poly <vilib>:"Read Key.vi"("section"=w998, "error in (no error)"=w992, "key"=w997, "refnum"=w995) -> ("error out"=w993:errorcluster, "value"=w999:path, "refnum out"=w994:T11)  [unwired: 4 in, 1 out]
                              n241 = property class="Ctl"(reference=w996, "Value"=w999) -> ()  [unwired: 1 in, 2 out]
                            }
                            frame "Cluster" {
                              w1009 = refnum<vi> refnum  # Cluster
                              n242 = To More Specific Class(target class=w1009, reference=w1007, error in=w1002) -> (specific class reference=w1008:refnum<vi>, error out=w1001:errorcluster)
                              n243 = property class="Clust"(reference=w1008, error in=w1001) -> (error out=w1000:errorcluster, "Label.Text"=w1005:string, "AllObjs[]"=w1006:refnum<vi>[])  [unwired: 1 out]
                              n244 = call "Final_Cluster_Key.vi"("AllObjs[]"=w1006, "error in (no error)"=w1000, "Label.Text"=w1005, "String"=w1003, "Refnum in"=w1004) -> ("error out"=w1010:errorcluster, "Refnum out"=w1011:T11)  [unwired: 5 in]
                            }
                            frame "I32" {
                              n245 = call-poly <vilib>:"Read Key.vi"("section"=w1018, "error in (no error)"=w1012, "key"=w1017, "refnum"=w1016) -> ("error out"=w1013:errorcluster, "value"=w1019:i32, "refnum out"=w1014:T11)  [unwired: 4 in, 1 out]
                              n246 = property class="Ctl"(reference=w1015, "Value"=w1019) -> ()  [unwired: 1 in, 2 out]
                            }
                            frame "U32" {
                              n247 = call-poly <vilib>:"Read Key.vi"("section"=w1026, "error in (no error)"=w1020, "key"=w1024, "refnum"=w1025) -> ("error out"=w1021:errorcluster, "value"=w1027:u32, "refnum out"=w1022:T11)  [unwired: 4 in, 1 out]
                              n248 = property class="Ctl"(reference=w1023, "Value"=w1027) -> ()  [unwired: 1 in, 2 out]
                            }
                            frame "U8" {
                              n249 = call-poly <vilib>:"Read Key.vi"("section"=w1034, "error in (no error)"=w1028, "key"=w1032, "refnum"=w1033) -> ("error out"=w1029:errorcluster, "value"=w1035:u32, "refnum out"=w1030:T11)  [unwired: 4 in, 1 out]
                              n250 = property class="Ctl"(reference=w1031, "Value"=w1035) -> ()  [unwired: 1 in, 2 out]
                            }
                            frame "Boolean" {
                              n251 = call-poly <vilib>:"Read Key.vi"("section"=w1042, "error in (no error)"=w1036, "key"=w1041, "refnum"=w1040) -> ("error out"=w1037:errorcluster, "value"=w1043:bool, "refnum out"=w1038:T11)  [unwired: 4 in, 1 out]
                              n252 = property class="Ctl"(reference=w1039, "Value"=w1043) -> ()  [unwired: 1 in, 2 out]
                            }
                            frame "Enum U8" {
                              n253 = call-poly <vilib>:"Read Key.vi"("section"=w1050, "error in (no error)"=w1044, "key"=w1048, "refnum"=w1049) -> ("error out"=w1045:errorcluster, "value"=w1051:u32, "refnum out"=w1046:T11)  [unwired: 4 in, 1 out]
                              n254 = property class="Ctl"(reference=w1047, "Value"=w1051) -> ()  [unwired: 1 in, 2 out]
                            }
                            frame "Refnum" {
                              n255 = call-poly <vilib>:"Read Key.vi"("section"=w1058, "error in (no error)"=w1052, "key"=w1057, "refnum"=w1056) -> ("error out"=w1053:errorcluster, "value"=w1059:string, "refnum out"=w1054:T11)  [unwired: 4 in, 1 out]
                              n256 = property class="Ctl"(reference=w1055, "Value"=w1059) -> ()  [unwired: 1 in, 2 out]
                            }
                          }
                        }
                      }
                      frame "I32" {
                        n257 = call-poly <vilib>:"Read Key.vi"("section"=w1066, "error in (no error)"=w1060, "key"=w1065, "refnum"=w1064) -> ("error out"=w1061:errorcluster, "value"=w1067:i32, "refnum out"=w1062:T11)  [unwired: 4 in, 1 out]
                        n258 = property class="Ctl"(reference=w1063, "Value"=w1067) -> ()  [unwired: 1 in, 2 out]
                      }
                      frame "U32" {
                        n259 = call-poly <vilib>:"Read Key.vi"("section"=w1074, "error in (no error)"=w1068, "key"=w1072, "refnum"=w1073) -> ("error out"=w1069:errorcluster, "value"=w1075:u32, "refnum out"=w1070:T11)  [unwired: 4 in, 1 out]
                        n260 = property class="Ctl"(reference=w1071, "Value"=w1075) -> ()  [unwired: 1 in, 2 out]
                      }
                      frame "U8" {
                        n261 = call-poly <vilib>:"Read Key.vi"("section"=w1082, "error in (no error)"=w1076, "key"=w1081, "refnum"=w1080) -> ("error out"=w1077:errorcluster, "value"=w1083:u32, "refnum out"=w1078:T11)  [unwired: 4 in, 1 out]
                        n262 = property class="Ctl"(reference=w1079, "Value"=w1083) -> ()  [unwired: 1 in, 2 out]
                      }
                      frame "Boolean" {
                        n263 = call-poly <vilib>:"Read Key.vi"("section"=w1090, "error in (no error)"=w1084, "key"=w1089, "refnum"=w1088) -> ("error out"=w1085:errorcluster, "value"=w1091:bool, "refnum out"=w1086:T11)  [unwired: 4 in, 1 out]
                        n264 = property class="Ctl"(reference=w1087, "Value"=w1091) -> ()  [unwired: 1 in, 2 out]
                      }
                      frame "Enum U8" {
                        n265 = call-poly <vilib>:"Read Key.vi"("section"=w1098, "error in (no error)"=w1092, "key"=w1096, "refnum"=w1097) -> ("error out"=w1093:errorcluster, "value"=w1099:u32, "refnum out"=w1094:T11)  [unwired: 4 in, 1 out]
                        n266 = property class="Ctl"(reference=w1095, "Value"=w1099) -> ()  [unwired: 1 in, 2 out]
                      }
                      frame "Refnum" {
                        n267 = call-poly <vilib>:"Read Key.vi"("section"=w1106, "error in (no error)"=w1100, "key"=w1105, "refnum"=w1104) -> ("error out"=w1101:errorcluster, "value"=w1107:string, "refnum out"=w1102:T11)  [unwired: 4 in, 1 out]
                        n268 = property class="Ctl"(reference=w1103, "Value"=w1107) -> ()  [unwired: 1 in, 2 out]
                      }
                    }
                  }
                }
                frame "I32" {
                  n269 = call-poly <vilib>:"Read Key.vi"("section"=w1114, "error in (no error)"=w1108, "key"=w1113, "refnum"=w1112) -> ("error out"=w1109:errorcluster, "value"=w1115:i32, "refnum out"=w1110:T11)  [unwired: 4 in, 1 out]
                  n270 = property class="Ctl"(reference=w1111, "Value"=w1115) -> ()  [unwired: 1 in, 2 out]
                }
                frame "U32" {
                  n271 = call-poly <vilib>:"Read Key.vi"("section"=w1122, "error in (no error)"=w1116, "key"=w1120, "refnum"=w1121) -> ("error out"=w1117:errorcluster, "value"=w1123:u32, "refnum out"=w1118:T11)  [unwired: 4 in, 1 out]
                  n272 = property class="Ctl"(reference=w1119, "Value"=w1123) -> ()  [unwired: 1 in, 2 out]
                }
                frame "U8" {
                  n273 = call-poly <vilib>:"Read Key.vi"("section"=w1130, "error in (no error)"=w1124, "key"=w1129, "refnum"=w1127) -> ("error out"=w1125:errorcluster, "value"=w1131:u32, "refnum out"=w1126:T11)  [unwired: 4 in, 1 out]
                  n274 = property class="Ctl"(reference=w1128, "Value"=w1131) -> ()  [unwired: 1 in, 2 out]
                }
                frame "Boolean" {
                  n275 = call-poly <vilib>:"Read Key.vi"("section"=w1138, "error in (no error)"=w1132, "key"=w1137, "refnum"=w1135) -> ("error out"=w1133:errorcluster, "value"=w1139:bool, "refnum out"=w1134:T11)  [unwired: 4 in, 1 out]
                  n276 = property class="Ctl"(reference=w1136, "Value"=w1139) -> ()  [unwired: 1 in, 2 out]
                }
                frame "Enum U8" {
                  n277 = call-poly <vilib>:"Read Key.vi"("section"=w1146, "error in (no error)"=w1140, "key"=w1144, "refnum"=w1145) -> ("error out"=w1141:errorcluster, "value"=w1147:u32, "refnum out"=w1142:T11)  [unwired: 4 in, 1 out]
                  n278 = property class="Ctl"(reference=w1143, "Value"=w1147) -> ()  [unwired: 1 in, 2 out]
                }
                frame "Refnum" {
                  n279 = call-poly <vilib>:"Read Key.vi"("section"=w1154, "error in (no error)"=w1148, "key"=w1153, "refnum"=w1152) -> ("error out"=w1149:errorcluster, "value"=w1155:string, "refnum out"=w1150:T11)  [unwired: 4 in, 1 out]
                  n280 = property class="Ctl"(reference=w1151, "Value"=w1155) -> ()  [unwired: 1 in, 2 out]
                }
              }
            }
          }
          frame "I32" {
            n281 = call-poly <vilib>:"Read Key.vi"("section"=w1162, "error in (no error)"=w1156, "key"=w1161, "refnum"=w1160) -> ("error out"=w1158:errorcluster, "value"=w1163:i32, "refnum out"=w1157:T11)  [unwired: 4 in, 1 out]
            n282 = property class="Ctl"(reference=w1159, "Value"=w1163) -> ()  [unwired: 1 in, 2 out]
          }
          frame "U32" {
            n283 = call-poly <vilib>:"Read Key.vi"("section"=w1170, "error in (no error)"=w1164, "key"=w1169, "refnum"=w1168) -> ("error out"=w1165:errorcluster, "value"=w1171:u32, "refnum out"=w1166:T11)  [unwired: 4 in, 1 out]
            n284 = property class="Ctl"(reference=w1167, "Value"=w1171) -> ()  [unwired: 1 in, 2 out]
          }
          frame "U8" {
            n285 = call-poly <vilib>:"Read Key.vi"("section"=w1178, "error in (no error)"=w1172, "key"=w1176, "refnum"=w1177) -> ("error out"=w1173:errorcluster, "value"=w1179:u32, "refnum out"=w1174:T11)  [unwired: 4 in, 1 out]
            n286 = property class="Ctl"(reference=w1175, "Value"=w1179) -> ()  [unwired: 1 in, 2 out]
          }
          frame "Boolean" {
            n287 = call-poly <vilib>:"Read Key.vi"("section"=w1186, "error in (no error)"=w1180, "key"=w1184, "refnum"=w1185) -> ("error out"=w1181:errorcluster, "value"=w1187:bool, "refnum out"=w1182:T11)  [unwired: 4 in, 1 out]
            n288 = property class="Ctl"(reference=w1183, "Value"=w1187) -> ()  [unwired: 1 in, 2 out]
          }
          frame "Enum U8" {
            n289 = call-poly <vilib>:"Read Key.vi"("section"=w1194, "error in (no error)"=w1188, "key"=w1192, "refnum"=w1193) -> ("error out"=w1189:errorcluster, "value"=w1195:u32, "refnum out"=w1190:T11)  [unwired: 4 in, 1 out]
            n290 = property class="Ctl"(reference=w1191, "Value"=w1195) -> ()  [unwired: 1 in, 2 out]
          }
          frame "Refnum" {
            n291 = call-poly <vilib>:"Read Key.vi"("section"=w1202, "error in (no error)"=w1196, "key"=w1201, "refnum"=w1200) -> ("error out"=w1197:errorcluster, "value"=w1203:string, "refnum out"=w1198:T11)  [unwired: 4 in, 1 out]
            n292 = property class="Ctl"(reference=w1199, "Value"=w1203) -> ()  [unwired: 1 in, 2 out]
          }
        }
      }
    }
    n293 = flat-sequence {
      tunnel: [w44] -> _
      tunnel: w30 -> [w44]
      tunnel: [w43] -> w29
      frame #0 {
        n294 = local read "Washer Variable"() -> (w43:T1)
      }
    }
  }
  "Output Cluster" <- w2
  n295 = local read "Local Control?"() -> (w7:bool)
  n296 = call <vilib>:"Close Config Data.vi"("error in (no error)"=w10, "refnum"=w9) -> ("error out"=w11:errorcluster)  [unwired: 8 in, 1 out]
  n297 = case shown="True" w7 {
    tunnel: w2 -> [_ w1204]
    frame False {
    }
    frame True {
      n298 = local write "Output Cluster"(w1204) -> ()
    }
  }
  n299 = flat-sequence {
    tunnel: w11 -> [w1205]
    frame #0 {
      "error out" <- w1205
    }
  }
